vi "MPM_imaging -v5.vi"() -> ()   [LabVIEW 2014]
uses:
  <vilib>/Analysis/baseanly.llb/Mean (DBL).vi
  <vilib>/DAQmx/read.llb/DAQmx Read (Analog 2D DBL NChan NSamp).vi
  <vilib>/DAQmx/read.llb/DAQmx Read (Analog 1D DBL 1Chan NSamp).vi
  <resource>/objmgr/daqmx.rc
  <vilib>/Analysis/NI_AALBase.lvlib
panel:
  out "Integratedfile":string
  out "Rawfile":string
  out "Standard deviationslow":dbl format="%.6f"
  out "Standard deviation fast":dbl format="%.6f"
  out "Mirror error":dbl[][](graph)
  out "Mirrors with offset":dbl[][](graph)
  out "Mirror position":dbl[][](graph)
  out "Samplenumbers":i32
  out "Delay (pixels)":dbl
  out "Galvo Delay (sec)":dbl format="%#_6e"
  out "Xrange":u16
  out "Execution time per loop":dbl[][](graph)
  out "Delay vs output":dbl[][](graph)
  in  "Index (col)":i32
  in  "Length to cut":i32
  in  "Delay increment":dbl=1e-07
  out "Execution time":dbl
  in  "No. of delay iterations":i32=1
  out "Delay vs output":dbl[][](array[numeric])
  out "ms timer":u32
  in  "Line scan on/off (raw)":bool
  in  "Line scan on/off (proccesed)":bool
  in  "Linear/log (integrated)":u16(ring) items=["linear", "log"]
  in  "Linecut direction (fast/slow) (integrated)":u16(ring) items=["fast", "slow"]
  out "Linecut profile (integrted)":dbl[](graph)
  out "Image (integrated)":dbl[][](graph)
  in  "error in (no error)":errorcluster
  out "error out":errorcluster
  out "Linecut profile (raw)":dbl[](graph)
  in  "Linear/Log (raw)":u16(ring) items=["Linear", "Log"]
  in  "Linecut direction (fast/slow) (raw)":u8(ring) items=["fast", "slow"]
  in  "Tab Control":enum32{"Scan and Image", "Save data"}(tab)
  out "Actual (sampling rate/pixel rate)":dbl
  in  "Soft reset after scan":bool
  out "Laser rep. rate (Hz)":dbl
  out "Actual (laser rep. rate/pixel rate)":dbl
  out "Actual pixel rate (Hz)":dbl
  out "Actual line scan rate (Hz)":dbl
  out "Initial sampling rate (Hz)":dbl
  in  "Scan dimension":T1(ring)
  in  "X scan parameters":T2={"Center \n"=0.0, "Scan amplitude"=1.0, "# of pixels"=100}
  in  "Y scan parameters":T3={"Center "=0.0, "Scan amplitude \n"=1.0, "# of pixels"=100}
  in  "Z scan parameters":T4
  out "Actual sampling rate (Hz)":dbl
  out "voltage/degree ratio (V/degree)":dbl
  in  "# of scans":u16(ring) items=["No scan", "Single scan", "Repeated scan"]
  in  "Initial line scan rate (Hz)":dbl(slide)=200.0 scale=0.0..200.0
  in  "Points/pixel":u16=6
  in  "+z":bool
  in  "-z":bool
  in  "Exit the program":bool
  in  "+x":bool
  in  "-x":bool
  in  "+y":bool
  in  "-y":bool
  out "Moving x":bool
  in  "X step":dbl=0.1
  in  "Move X":dbl=14.3034736
  out "Moving y":bool
  in  "Y step":dbl=1.0
  in  "Move Y":dbl=11.6422302
  out "upper z-limit":dbl
  out "lower z-limit":dbl
  out "Moving z":bool
  in  "Z step":dbl=0.001
  in  "Move Z":dbl=18.8888872
  in  "set lower z-limit":dbl
  in  "set upper z-limit":dbl=19.2
  in  "Average in other dim":dbl=1.0
  out "z stack":i32
  out "single (line counter)":i32
  out "Frame rate (s)":dbl format="%.4f"
  out "Time left for stack (s)":dbl format="%#.2g"
  out "lower y-limit":dbl
  out "upper y-limit":dbl
  out "lower x-limit":dbl
  out "upper x-limit":dbl
  in  "set upper y-limit":dbl
  in  "set lower y-limit":dbl
  in  "set upper x-limit":dbl
  in  "set lower x-limit":dbl
  in  "Row by row update?":bool=TRUE
  in  "Stop":bool
  in  "Sample clock source":tag="/Dev1/PFI0"
  in  "Scan mode":T5(ring)=enum."Single Direction (Uniform)"
  out "Theoretical frame rate":dbl format="%_5g"
  in  "Galvomirror delay (sec)":dbl=0.0003 format="%#_6e"
  in  "Lissajous Cluster":cluster{"a":dbl, "b":dbl, "delta":dbl}={"a"=1.0, "b"=2.0, "delta"=0.0} {"delta" format="%_3g"; "b" format="%0.2p"; "a" format="%_3g"}
  in  "Laser rep rate":dbl=120000.0 format="%#_13g"
  out "Galvo speed OK?":bool
  out "Onboard Sample clock?":bool
  in  "Soften":bool
  in  "Asymmetry sawtooth":dbl=0.5
  in  "Sample Clock Delay":dbl=6.7e-06
  in  "Delay from sample clock":bool
  in  "Samp Clk. Delay Units":i32(ring)=10364 items=["Seconds"=10364, "Ticks"=10304]
  in  "Soften points":i32=3
  in  "Track mirror":bool
  out "Pixel Delay":dbl
  in  "File name (integrated). (must end with extension \".txt\")":string="run1_p.txt"
  out "Appended path (integrated)":path
  out "Save tiff stack (integrated)?":bool=TRUE
  out "Auto-save during single scan (integrated)?":bool=TRUE
  out "Save tiff stack (raw)?":bool
  in  "Auto-save during single scan (raw)?":bool=TRUE
  in  "File name (raw). (must end with extension \".txt\")":string="run1_r.txt"
  out "Appended path (raw)":path
  out "Image (raw)":dbl[][](graph)
  # "Controls"
  # "Galvo tracking and\ndelay compensation"
  # "piezo:      0-20   um   \ngalvo: -10 - 10 degrees"
  # "piezo:      0-20   um   \ngalvo: -10 - 10 degrees"
  # "piezo:      0-20   um   \ngalvo: -10 - 10 degrees"
  # "Move sample stage"
  # "Smoothening parameters"
  # "Pattern parameters"
  # "Trigger Delay parameters"
  # "Indicators"
  # "(only for galvomirrors)"
  # "(>=2 when pixel rate is lower than amplifier bandwidth)"
  # "(>=10 )"
  # "(piezo: um/galvo: degree)"
  # "(piezo: um/galvo: degree)"
  # "(>1)"
  # "(piezo: um/galvo: degree)"
  # "(piezo: um/galvo: degree)"
  # "(>1)"
  # "(piezo: um/galvo: degree)"
  # "(piezo: um/galvo: degree)"
  # "(>1)"
  # "Raw"
  # "Pixel integrated"
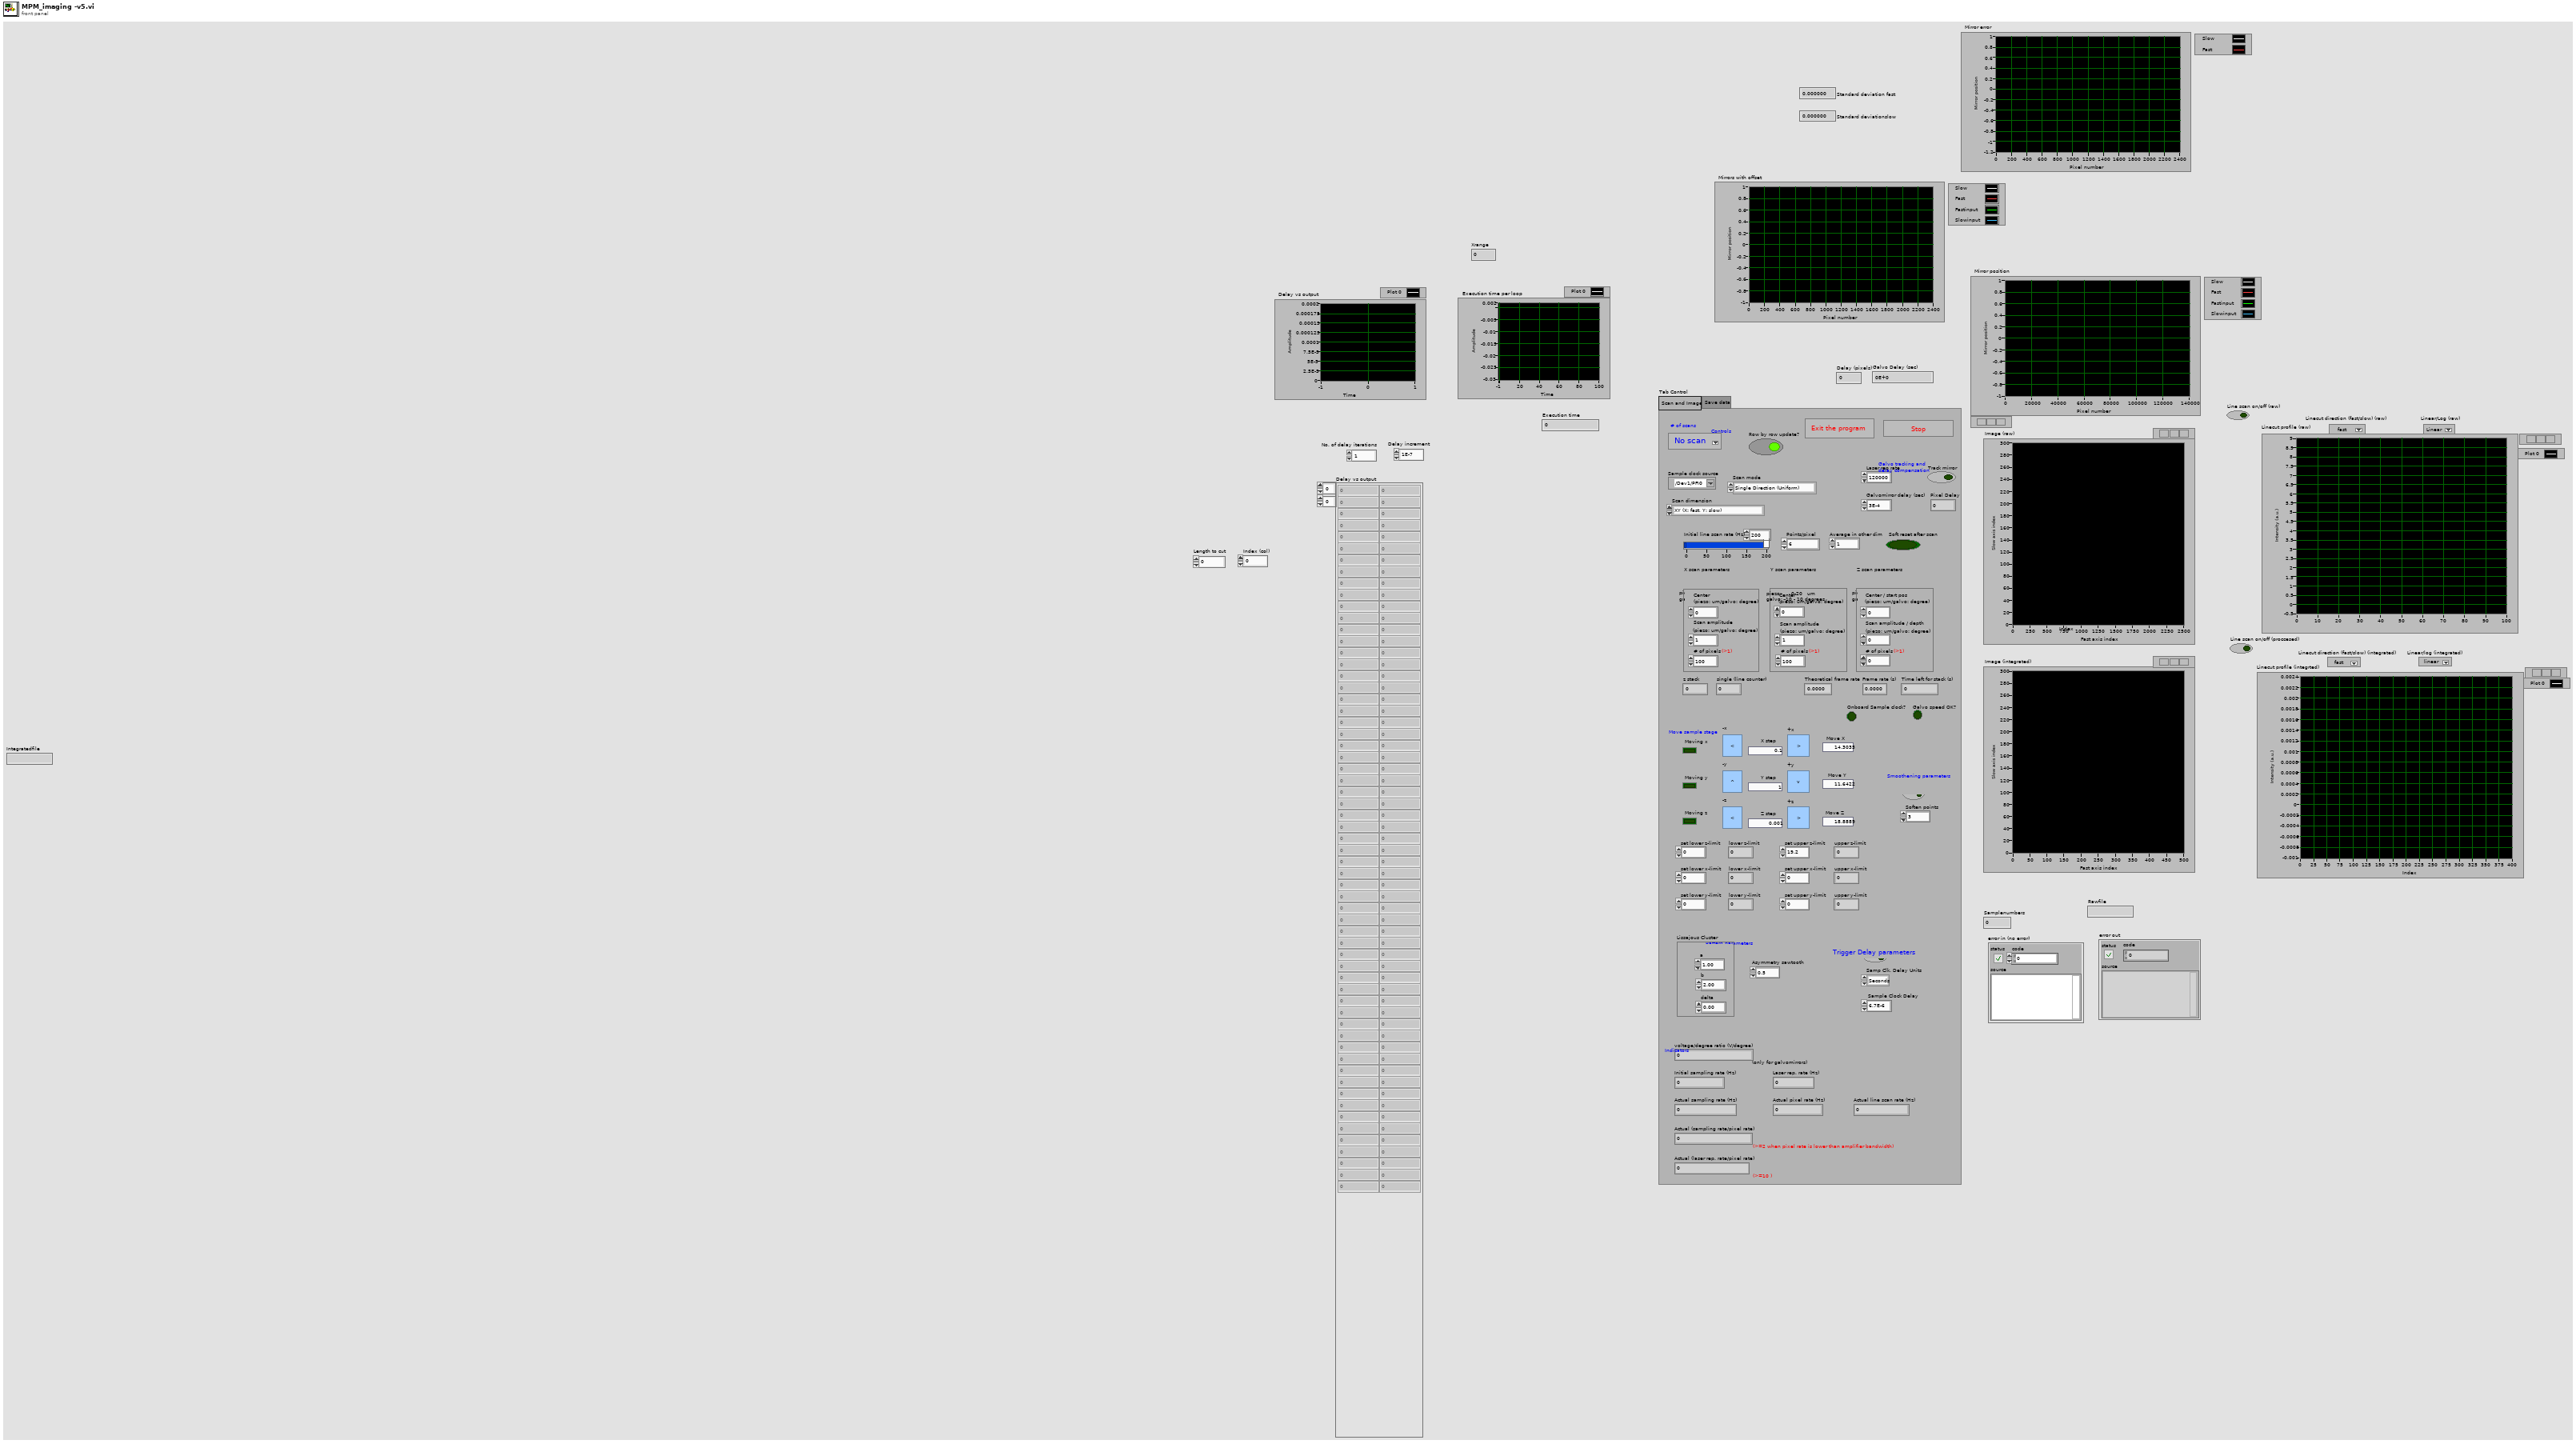
[diagram p1: front panel]
types:
  T1 = enum8{"XY (X: fast, Y: slow)", "XYZ (X: fast, Y: medium, Z: slow)"}
  T2 = cluster{"Center \n":dbl, "Scan amplitude":dbl, "# of pixels":u16}
  T3 = cluster{"Center ":dbl, "Scan amplitude \n":dbl, "# of pixels":u16}
  T4 = cluster{"Center / start pos ":dbl, "Scan amplitude / depth\n":dbl, "# of pixels":u16}
  T5 = enum16{"Lissajous", "Adjustable sawtooth", "Single Direction (Uniform)", "Single Direction (Fast Reset)", "Bi-Directional"}
  T6 = cluster{"VISA resource name":refnum<visa-resource-name>, "Device name":string, "Controller address":i32, "error":errorcluster}
  T7 = cluster{"# of pixels":u16, "Center / start pos ":dbl, "Scan amplitude / depth\n":dbl}
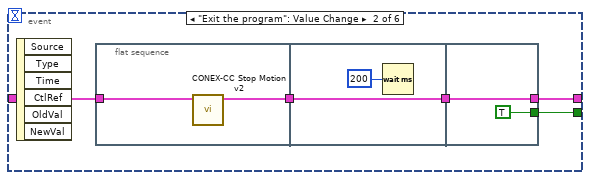
[diagram p2: hidden frame]
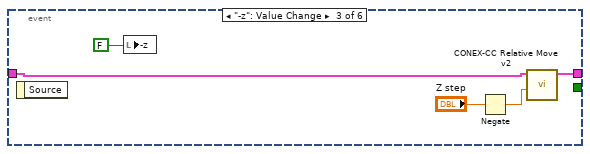
[diagram p3: hidden frame]
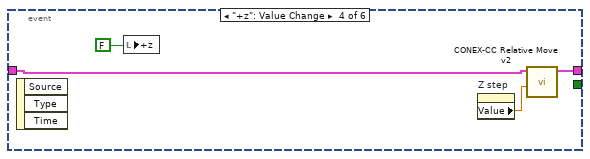
[diagram p4: hidden frame]
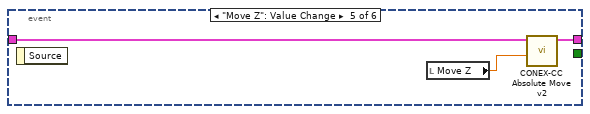
[diagram p5: hidden frame]
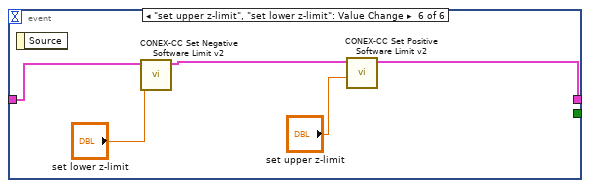
[diagram p6: hidden frame]
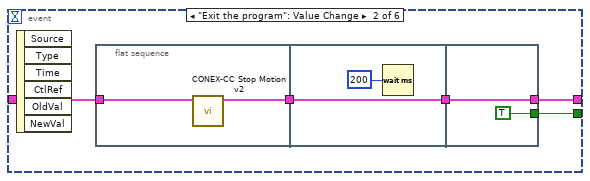
[diagram p7: hidden frame]
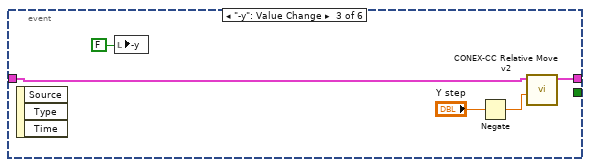
[diagram p8: hidden frame]
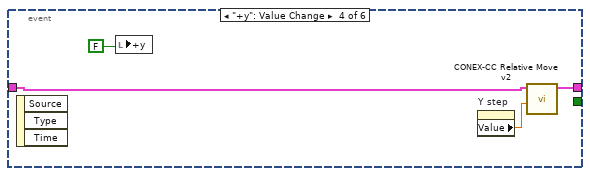
[diagram p9: hidden frame]
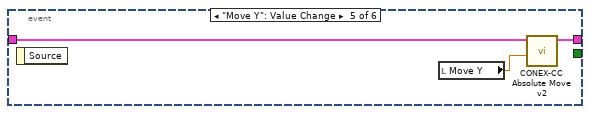
[diagram p10: hidden frame]
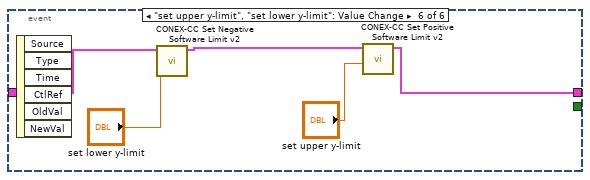
[diagram p11: hidden frame]
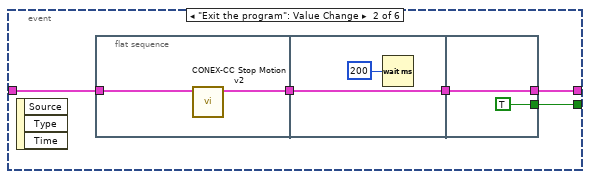
[diagram p12: hidden frame]
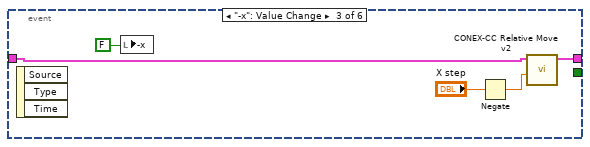
[diagram p13: hidden frame]
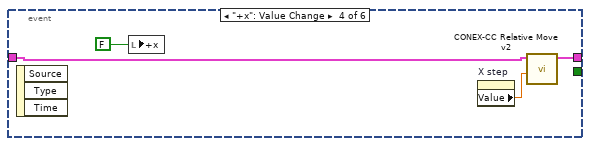
[diagram p14: hidden frame]
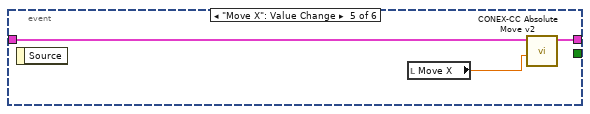
[diagram p15: hidden frame]
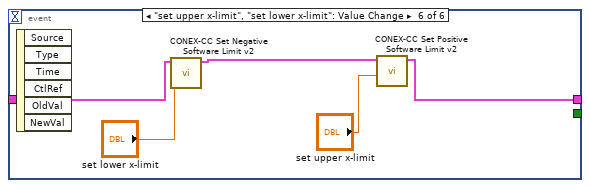
[diagram p16: hidden frame]
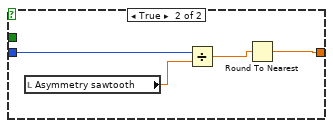
[diagram p18: hidden frame]
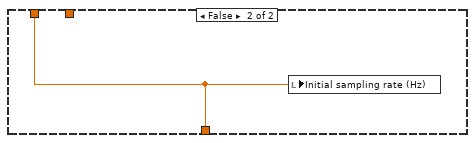
[diagram p19: hidden frame]
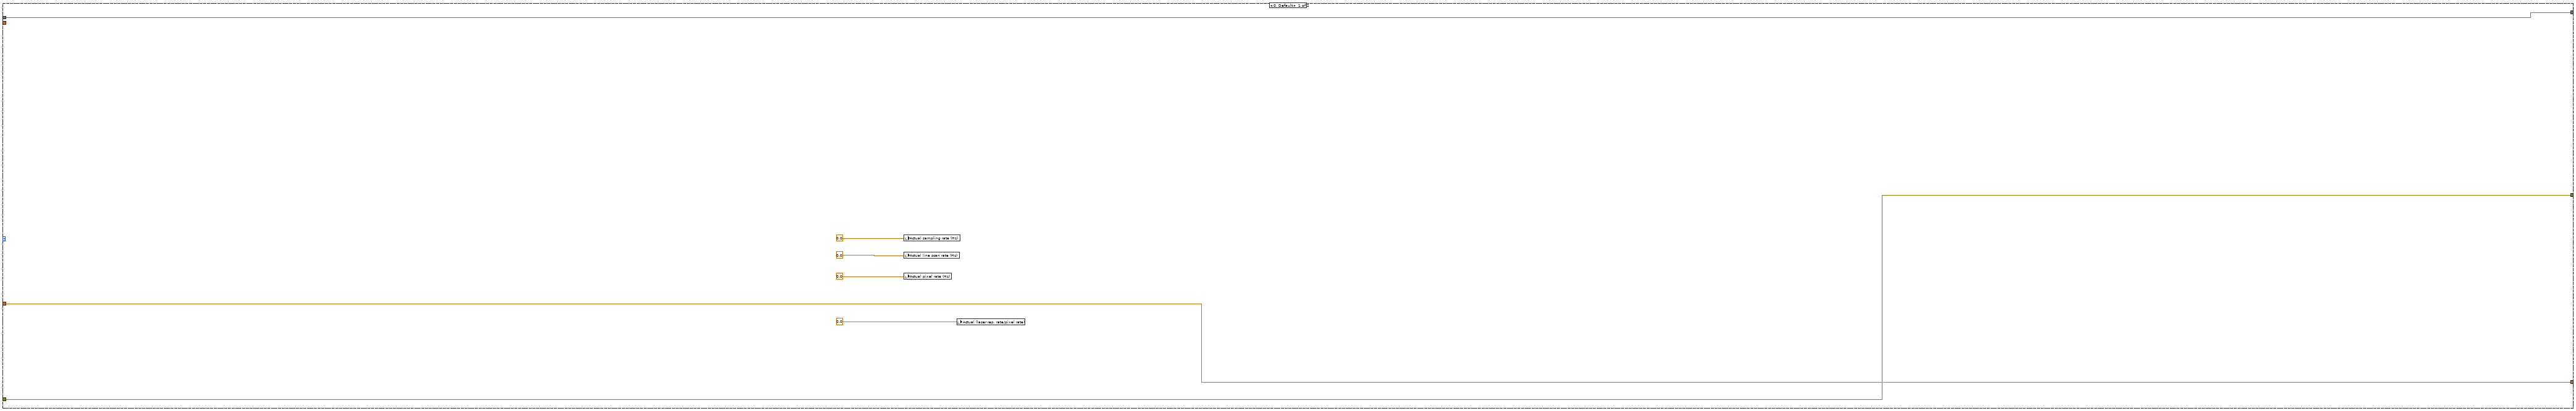
[diagram p20: hidden frame]
diagram:
  w14 = FALSE
  # "There is a physical delay of galvo response (Small Angle Step Response of around 3 microsec) which can be verified in the track mirror option (given by Galvo Delay (sec) and Delay (Pixels)).\nThis delay can be included while taking images in the control 'Galvomirror delay'.  \nGalvomirror delay x  initial sampling rate (laser rep rate for laser as trigger) is the correspong delay in pixel number."
  # "Adjustable sawtooth pattern is controlled by asymmetry sawtooth control. When it is 0.5 the pattern is a triangle. For asymmetry sawtooth =0.9 the pattern becomes single\ndirection fast reset"
  # "Soften is for smoothening the raster pattern.  Twice the number of soften points are added both at the peak and dip. This means in one fast axis cycle 4 x soften points are added."
  # "Sample clock delay is the delay between fluoresecence peak and laser trigger (when sample clock is laser trigger). This delay is varied from 1E-7 (can't be zero) to 8 microsec  in a loop which runs 'no. of delay iterations' times to obtain the maximum signal. The delay is then set to that value.  Delay value depends only on the pre-amp settings and in general lies between 6.8E-6 to 7.5E-6"
  # "0: no scan, 1: single scan, 2: repeat scan"
  # "Newport controls"
  # "only for galvomirrors"
  # "piezo:      0-20   um   \ngalvo: -10 - 10 degrees"
  # "piezo:      0-20   um   \ngalvo: -10 - 10 degrees"
  # "piezo:      0-20   um   \ngalvo: -10 - 10 degrees"
  n1 = local write "-x"(w14) -> ()
  n2 = local write "+x"(w14) -> ()
  n3 = Format Date/Time String(time format string (%c)="%H_%M_%S_") -> (date/time string=w3:string)  [unwired: 2 in]
  n4 = Format Date/Time String(time format string (%c)="%H_%M_%S_") -> (date/time string=w7:string)  [unwired: 2 in]
  n5 = Concatenate Strings(w3, "File name (integrated). (must end with extension \".txt\")") -> (→"Integratedfile":string)
  n6 = call "Connect Newport Instrument_edit.vi"("Numeric"=i8 1, "String"="ASRL4::INSTR") -> ("Device Connection Cluster"=w16:T6)  [unwired: 5 in, 4 out]
  n7 = call "Connect Newport Instrument_edit.vi"("Numeric"=i8 1, "String"="ASRL3::INSTR") -> ("Device Connection Cluster"=w15:T6)  [unwired: 5 in, 4 out]
  n8 = call "Connect Newport Instrument_edit.vi"("Numeric"=i8 1, "String"="ASRL5::INSTR") -> ("Device Connection Cluster"=w9:T6)  [unwired: 5 in, 4 out]
  n9 = Concatenate Strings(w7, "File name (raw). (must end with extension \".txt\")") -> (→"Rawfile":string)
  n10 = while {
    shift-right: [w32] -> w12
    shift-left: w16 -> [w31]
    stop <- w30 stop-if-true
    n11 = event shown="[0] Timeout" {
      selector: _ -> [_ _ _ _ _ _]
      dyn-events: _ -> [_ _ _ _ _ _]
      timeout: 100 -> [_ _ _ _ _ _]
      tunnel: [_ w46 _ _ _ _] -> w30
      tunnel: w31 -> [w44 w47 w57 w63 w67 w69]
      tunnel: [w43 w49 w60 w62 w66 w68] -> w32
      event Timeout {
        n12 = event-data() -> ()  [unwired: 4 out]
        n13 = call "CONEX-CC Get Current Position v2.vi"("Connection Cluster in"=w44) -> ("Current position"=w38:dbl, "Connection Cluster out"=w37:T6)  [unwired: 8 in, 1 out]
        n14 = local write "Move Y"(w38) -> ()
        n15 = Unbundle By Name(w37) -> ("error"=w39:errorcluster)  [unwired: 1 out]
        n16 = call "CONEX-CC Get Negative Software Limit v2.vi"("Connection Cluster in"=w37) -> ("Left limit"=→"lower y-limit":dbl, "Connection Cluster out"=w36:T6)  [unwired: 9 in]
        n17 = call "CONEX-CC Get Positive Software Limit v2.vi"("Connection Cluster in"=w36) -> ("Right limit"=→"upper y-limit":dbl, "Connection Cluster out"=w35:T6)  [unwired: 9 in]
        n18 = local write "error out"(w39) -> ()
        n19 = call "CONEX-CC Get Positioner Error And Controller State v2.vi"("Connection Cluster in"=w35) -> ("Controller state"=w42:string, "Connection Cluster out"=w43:T6)  [unwired: 8 in, 1 out]
        n20 = Equal?(x="28" ("y"), y=w42) -> (x = y?=→"Moving y":bool)
      }
      event "Exit the program": Value Change {
        n21 = event-data() -> ()  [unwired: 7 out]
        n22 = flat-sequence {
          tunnel: [w51] -> w45
          tunnel: w47 -> [w50]
          tunnel: w45 -> [w53]
          tunnel: [w53] -> w48
          tunnel: [w55] -> w49
          tunnel: w48 -> [w55]
          tunnel: [TRUE] -> w46
          frame #0 {
            n23 = call "CONEX-CC Stop Motion v2.vi"("Connection Cluster in"=w50) -> ("Connection Cluster out"=w51:T6)  [unwired: 10 in]
          }
          frame #1 {
            n24 = Wait (ms)(milliseconds to wait=u32 200 ("attente (ms)")) -> ()  [unwired: 1 out]
          }
          frame #2 {
          }
        }
      }
      event "-y": Value Change {
        n25 = event-data() -> ()  [unwired: 4 out]
        n26 = local write "-y"(FALSE ("-")) -> ()
        n27 = Negate(x="Y step") -> (-x=w58:dbl)
        n28 = call "CONEX-CC Relative Move v2.vi"("Relative displacement"=w58, "Connection Cluster in"=w57) -> ("Connection Cluster out"=w60:T6)  [unwired: 9 in]
      }
      event "+y": Value Change {
        n29 = event-data() -> ()  [unwired: 4 out]
        n30 = local write "+y"(FALSE ("+")) -> ()
        n31 = property on="Y step" class="DigNum (strict)"() -> ("Value"=w64:dbl)  [unwired: 2 in, 2 out]
        n32 = call "CONEX-CC Relative Move v2.vi"("Relative displacement"=w64, "Connection Cluster in"=w63) -> ("Connection Cluster out"=w62:T6)  [unwired: 9 in]
      }
      event "Move Y": Value Change {
        n33 = event-data() -> ()  [unwired: 2 out]
        n34 = local read "Move Y"() -> (w65:dbl)
        n35 = call "CONEX-CC Absolute Move v2.vi"("Target position"=w65, "Connection Cluster in"=w67) -> ("Connection Cluster out"=w66:T6)  [unwired: 5 in, 2 out]
      }
      event "set upper y-limit", "set lower y-limit": Value Change {
        n36 = event-data() -> ()  [unwired: 7 out]
        n37 = call "CONEX-CC Set Negative Software Limit v2.vi"("Negative limit (left)"="set lower y-limit", "Connection Cluster in"=w69) -> ("Connection Cluster out"=w72:T6)  [unwired: 9 in]
        n38 = call "CONEX-CC Set Positive Software Limit v2.vi"("Positive limit (right)"="set upper y-limit", "Connection Cluster in"=w72) -> ("Connection Cluster out"=w68:T6)  [unwired: 9 in]
      }
    }
  }
  n39 = while {
    shift-right: [w76] -> w11
    shift-left: w9 -> [w75]
    stop <- w74 stop-if-true
    n40 = event shown="[0] Timeout" {
      selector: _ -> [_ _ _ _ _ _]
      dyn-events: _ -> [_ _ _ _ _ _]
      timeout: 100 -> [_ _ _ _ _ _]
      tunnel: [_ w90 _ _ _ _] -> w74
      tunnel: w75 -> [w88 w91 w101 w107 w111 w116]
      tunnel: [w87 w93 w104 w106 w110 w114] -> w76
      event Timeout {
        n41 = event-data() -> ()  [unwired: 4 out]
        n42 = call "CONEX-CC Get Current Position v2.vi"("Connection Cluster in"=w88) -> ("Current position"=w77:dbl, "Connection Cluster out"=w83:T6)  [unwired: 8 in, 1 out]
        n43 = local write "Move Z"(w77) -> ()
        n44 = Unbundle By Name(w83) -> ("error"=w78:errorcluster)  [unwired: 1 out]
        n45 = call "CONEX-CC Get Negative Software Limit v2.vi"("Connection Cluster in"=w83) -> ("Left limit"=→"lower z-limit":dbl, "Connection Cluster out"=w82:T6)  [unwired: 9 in]
        n46 = call "CONEX-CC Get Positive Software Limit v2.vi"("Connection Cluster in"=w82) -> ("Right limit"=→"upper z-limit":dbl, "Connection Cluster out"=w81:T6)  [unwired: 9 in]
        n47 = local write "error out"(w78) -> ()
        n48 = call "CONEX-CC Get Positioner Error And Controller State v2.vi"("Connection Cluster in"=w81) -> ("Controller state"=w86:string, "Connection Cluster out"=w87:T6)  [unwired: 8 in, 1 out]
        n49 = Equal?(x=w86, y="28") -> (x = y?=→"Moving z":bool)
      }
      event "Exit the program": Value Change {
        n50 = event-data() -> ()  [unwired: 7 out]
        n51 = flat-sequence {
          tunnel: [w95] -> w89
          tunnel: w91 -> [w94]
          tunnel: w89 -> [w97]
          tunnel: [w97] -> w92
          tunnel: [w99] -> w93
          tunnel: w92 -> [w99]
          tunnel: [TRUE] -> w90
          frame #0 {
            n52 = call "CONEX-CC Stop Motion v2.vi"("Connection Cluster in"=w94) -> ("Connection Cluster out"=w95:T6)  [unwired: 10 in]
          }
          frame #1 {
            n53 = Wait (ms)(milliseconds to wait=u32 200 ("attente (ms)")) -> ()  [unwired: 1 out]
          }
          frame #2 {
          }
        }
      }
      event "-z": Value Change {
        n54 = event-data() -> ()  [unwired: 2 out]
        n55 = local write "-z"(FALSE ("-")) -> ()
        n56 = Negate(x="Z step") -> (-x=w102:dbl)
        n57 = call "CONEX-CC Relative Move v2.vi"("Relative displacement"=w102, "Connection Cluster in"=w101) -> ("Connection Cluster out"=w104:T6)  [unwired: 9 in]
      }
      event "+z": Value Change {
        n58 = event-data() -> ()  [unwired: 4 out]
        n59 = local write "+z"(FALSE ("+")) -> ()
        n60 = property on="Z step" class="DigNum (strict)"() -> ("Value"=w108:dbl)  [unwired: 2 in, 2 out]
        n61 = call "CONEX-CC Relative Move v2.vi"("Relative displacement"=w108, "Connection Cluster in"=w107) -> ("Connection Cluster out"=w106:T6)  [unwired: 9 in]
      }
      event "Move Z": Value Change {
        n62 = event-data() -> ()  [unwired: 2 out]
        n63 = local read "Move Z"() -> (w109:dbl)
        n64 = call "CONEX-CC Absolute Move v2.vi"("Target position"=w109, "Connection Cluster in"=w111) -> ("Connection Cluster out"=w110:T6)  [unwired: 5 in, 2 out]
      }
      event "set upper z-limit", "set lower z-limit": Value Change {
        n65 = event-data() -> ()  [unwired: 2 out]
        n66 = call "CONEX-CC Set Negative Software Limit v2.vi"("Negative limit (left)"="set lower z-limit", "Connection Cluster in"=w116) -> ("Connection Cluster out"=w115:T6)  [unwired: 9 in]
        n67 = call "CONEX-CC Set Positive Software Limit v2.vi"("Positive limit (right)"="set upper z-limit", "Connection Cluster in"=w115) -> ("Connection Cluster out"=w114:T6)  [unwired: 9 in]
      }
    }
  }
  n68 = while {
    shift-right: [w120] -> w13
    shift-left: w15 -> [w119]
    stop <- w118 stop-if-true
    n69 = event shown="[0] Timeout" {
      selector: _ -> [_ _ _ _ _ _]
      dyn-events: _ -> [_ _ _ _ _ _]
      timeout: 100 -> [_ _ _ _ _ _]
      tunnel: [_ w134 _ _ _ _] -> w118
      tunnel: w119 -> [w132 w135 w145 w151 w155 w157]
      tunnel: [w131 w137 w148 w150 w154 w156] -> w120
      event Timeout {
        n70 = event-data() -> ()  [unwired: 4 out]
        n71 = call "CONEX-CC Get Current Position v2.vi"("Connection Cluster in"=w132) -> ("Current position"=w126:dbl, "Connection Cluster out"=w125:T6)  [unwired: 8 in, 1 out]
        n72 = local write "Move X"(w126) -> ()
        n73 = Unbundle By Name(w125) -> ("error"=w127:errorcluster)  [unwired: 1 out]
        n74 = call "CONEX-CC Get Negative Software Limit v2.vi"("Connection Cluster in"=w125) -> ("Left limit"=→"lower x-limit":dbl, "Connection Cluster out"=w124:T6)  [unwired: 9 in]
        n75 = call "CONEX-CC Get Positive Software Limit v2.vi"("Connection Cluster in"=w124) -> ("Right limit"=→"upper x-limit":dbl, "Connection Cluster out"=w123:T6)  [unwired: 9 in]
        n76 = local write "error out"(w127) -> ()
        n77 = call "CONEX-CC Get Positioner Error And Controller State v2.vi"("Connection Cluster in"=w123) -> ("Controller state"=w130:string, "Connection Cluster out"=w131:T6)  [unwired: 8 in, 1 out]
        n78 = Equal?(x=w130, y="28") -> (x = y?=→"Moving x":bool)
      }
      event "Exit the program": Value Change {
        n79 = event-data() -> ()  [unwired: 4 out]
        n80 = flat-sequence {
          tunnel: [w139] -> w133
          tunnel: w135 -> [w138]
          tunnel: w133 -> [w141]
          tunnel: [w141] -> w136
          tunnel: [w143] -> w137
          tunnel: w136 -> [w143]
          tunnel: [TRUE] -> w134
          frame #0 {
            n81 = call "CONEX-CC Stop Motion v2.vi"("Connection Cluster in"=w138) -> ("Connection Cluster out"=w139:T6)  [unwired: 10 in]
          }
          frame #1 {
            n82 = Wait (ms)(milliseconds to wait=u32 200 ("attente (ms)")) -> ()  [unwired: 1 out]
          }
          frame #2 {
          }
        }
      }
      event "-x": Value Change {
        n83 = event-data() -> ()  [unwired: 4 out]
        n84 = local write "-x"(FALSE ("-")) -> ()
        n85 = Negate(x="X step") -> (-x=w146:dbl)
        n86 = call "CONEX-CC Relative Move v2.vi"("Relative displacement"=w146, "Connection Cluster in"=w145) -> ("Connection Cluster out"=w148:T6)  [unwired: 9 in]
      }
      event "+x": Value Change {
        n87 = event-data() -> ()  [unwired: 4 out]
        n88 = local write "+x"(FALSE ("+")) -> ()
        n89 = property on="X step" class="DigNum (strict)"() -> ("Value"=w152:dbl)  [unwired: 2 in, 2 out]
        n90 = call "CONEX-CC Relative Move v2.vi"("Relative displacement"=w152, "Connection Cluster in"=w151) -> ("Connection Cluster out"=w150:T6)  [unwired: 9 in]
      }
      event "Move X": Value Change {
        n91 = event-data() -> ()  [unwired: 2 out]
        n92 = local read "Move X"() -> (w153:dbl)
        n93 = call "CONEX-CC Absolute Move v2.vi"("Target position"=w153, "Connection Cluster in"=w155) -> ("Connection Cluster out"=w154:T6)  [unwired: 5 in, 2 out]
      }
      event "set upper x-limit", "set lower x-limit": Value Change {
        n94 = event-data() -> ()  [unwired: 7 out]
        n95 = call "CONEX-CC Set Negative Software Limit v2.vi"("Negative limit (left)"="set lower x-limit", "Connection Cluster in"=w157) -> ("Connection Cluster out"=w160:T6)  [unwired: 9 in]
        n96 = call "CONEX-CC Set Positive Software Limit v2.vi"("Positive limit (right)"="set upper x-limit", "Connection Cluster in"=w160) -> ("Connection Cluster out"=w156:T6)  [unwired: 9 in]
      }
    }
  }
  n97 = while {
    tunnel: w9 -> [w200]
    tunnel: [w199] -> w10
    stop <- "Exit the program" stop-if-true
    # "For Case II above clock sampling rate is independent of initial line\nscan rate. Laser rep rate is the sampling rate."
    # "a:  Laser rep rate: points/sec\nb:  X scan #of pixels x points/pixel: points/line\nCase I: When sample clock source is the laser trigger\nline scan rate is a/b which should always be less than 200 Hz\n(maximum freq. of galvo)\nTherefore b > laser rep rate/200\nCase II: When sample clock source is DAQ onboard clock, the galvo freq.\nis independent of laser rep. rate and ia given by initial line scan rate\n(set by user with maximum value as 200)"
    # "Maximum galvo rate"
    # "Actual line scan rate \nwith laser trigger as sample clock"
    n98 = local read "X scan parameters"() -> (w186:T2)
    n99 = local read "Scan mode"() -> (w166:T5)
    n100 = Unbundle By Name(w186) -> ("# of pixels"=w163:u16)
    n101 = Equal?(x=w166, y=T5."Adjustable sawtooth") -> (x = y?=w164:bool)
    n102 = Equal?(x=w166, y=T5."Single Direction (Fast Reset)") -> (x = y?=w161:bool)
    n103 = case shown="False" w164 {
      tunnel: w163 -> [w202 w211]
      tunnel: [w201 w209] -> w162
      tunnel: w161 -> [w203 _]
      frame False {
        n104 = case shown="True" w203 {
          tunnel: w202 -> [w204 w207]
          tunnel: [w204 w205] -> w201
          frame False {
          }
          frame True {
            n105 = Divide(x=w207, y=0.9) -> (x/y=w206:dbl)
            n106 = Round To Nearest(number=w206) -> (nearest integer value=w205:dbl)
          }
        }
      }
      frame True {
        n107 = local read "Asymmetry sawtooth"() -> (w212:dbl)
        n108 = Divide(x=w211, y=w212) -> (x/y=w210:dbl)
        n109 = Round To Nearest(number=w210) -> (nearest integer value=w209:dbl)
      }
    }
    n110 = local read "Onboard Sample clock?"() -> (w176:bool)
    n111 = local read "error in (no error)"() -> (w174:errorcluster)
    n112 = local read "Initial sampling rate (Hz)"() -> (w168:dbl)
    n113 = local write "Sample Clock Delay"("Sample Clock Delay") -> ()
    n114 = local read "Sample clock source"() -> (w188:tag)
    n115 = local read "Points/pixel"() -> (w187:u16)
    n116 = Multiply(x=w187, y=w162) -> (x*y=w177:dbl)
    n117 = case shown="True" w176 {
      tunnel: w177 -> [w215 _]
      tunnel: "Laser rep rate" -> [_ w216]
      tunnel: [w213 w216] -> w172
      frame True {
        n118 = local read "Initial line scan rate (Hz)"() -> (w214:dbl)
        n119 = Multiply(x=w215, y=w214) -> (x*y=w213:dbl)
        n120 = local write "Initial sampling rate (Hz)"(w213) -> ()
      }
      frame False {
        n121 = local write "Initial sampling rate (Hz)"(w216) -> ()
      }
    }
    n122 = Not Equal?(x=w188, y=tag "/Dev1/PFI0") -> (x != y?=w179:bool)
    "Onboard Sample clock?" <- w179
    n123 = Divide(x=w168, y=w177) -> (x/y=w180:dbl)
    n124 = local read "Y scan parameters"() -> (w185:T3)
    n125 = Divide(x="Laser rep rate", y=ext 200.0) -> (x/y=w181:ext)
    n126 = Greater Or Equal?(x=w177, y=w181) -> (x >= y?=w178:bool)
    n127 = Reciprocal(x=w172) -> (1/x=w170:dbl)
    n128 = Unbundle By Name(w185) -> ("# of pixels"=w184:u16)
    n129 = Or(x=w179, y=w178) -> (x .or. y?=→"Galvo speed OK?":bool)
    n130 = Divide(x="Galvomirror delay (sec)", y=w170) -> (x/y=→"Pixel Delay":dbl)
    n131 = Divide(x=w184, y=w180) -> (x/y=→"Theoretical frame rate":dbl)
    n132 = Initialize Array(0.0 ("element"), 100 ("dimension size"), 2 ("dimension size")) -> (w193:dbl[][])
    n133 = for {
      N: "No. of delay iterations" -> [_]
      tunnel: w174 -> [w228]
      tunnel: w200 -> [w225]
      tunnel: [w224] -> w199
      shift-right: [w220] -> _
      shift-left: "Sample Clock Delay" -> [w219]
      tunnel: [w223] -> _ mode=indexing
      tunnel: w193 -> [w223] mode=indexing
      tunnel: [w222] -> w192 mode=indexing
      n134 = call "Time Delay"("error in (no error)"=w228, "Delay Time (s)"=0.1) -> ("error out"=w227:errorcluster)  [unwired: 9 in]
      n135 = local read "# of scans"() -> (w229:u16)
      n136 = case shown="1, 2" w229 {
        tunnel: w227 -> [w236 w267]
        tunnel: [w236 w256] -> w224
        tunnel: w225 -> [_ w260]
        tunnel: w219 -> [w231 w246]
        tunnel: [w231 w252] -> w218
        tunnel: w223 -> [w230 w251]
        tunnel: w219 -> [_ w250]
        tunnel: [w230 w249] -> w222
        tunnel: "Stop" -> [_ w245]
        frame 0, Default {
          n137 = local write "Actual sampling rate (Hz)"(0.0) -> ()
          n138 = local write "Actual line scan rate (Hz)"(0.0) -> ()
          n139 = local write "Actual pixel rate (Hz)"(0.0) -> ()
          n140 = local write "Actual (laser rep. rate/pixel rate)"(0.0) -> ()
        }
        frame 1, 2 {
          w274 = 1.0
          n141 = local read "Y scan parameters"() -> (w280:T3)
          n142 = local read "Scan mode"() -> (w241:T5)
          n143 = local read "X scan parameters"() -> (w285:T2)
          n144 = local read "Z scan parameters"() -> (w275:T4)
          n145 = local write "voltage/degree ratio (V/degree)"(w274) -> ()
          n146 = Unbundle By Name(w275) -> ("Center / start pos"=w261:dbl, "Scan amplitude / depth"=w247:dbl, "# of pixels"=w268:u16)
          n147 = Unbundle By Name(w280) -> ("Center"=w279:dbl, "Scan amplitude"=w278:dbl, "# of pixels"=w269:u16)
          n148 = Unbundle By Name(w285) -> ("Center"=w284:dbl, "Scan amplitude"=w283:dbl, "# of pixels"=w242:u16)
          n149 = Equal?(x=w241, y=T5."Adjustable sawtooth") -> (x = y?=w243:bool)
          n150 = Equal?(x=w241, y=T5."Single Direction (Fast Reset)") -> (x = y?=w239:bool)
          n151 = case shown="True" w243 {
            tunnel: w242 -> [w287 w295]
            tunnel: [w286 w293] -> w238
            tunnel: w239 -> [w288 _]
            frame False {
              n152 = case shown="False" w288 {
                tunnel: w287 -> [w289 w291]
                tunnel: [w289 w290] -> w286
                frame False {
                }
                frame True {
                  n153 = Divide(x=w291, y=0.9) -> (x/y=w290:dbl)
                }
              }
            }
            frame True {
              n154 = local read "Asymmetry sawtooth"() -> (w294:dbl)
              n155 = Divide(x=w295, y=w294) -> (x/y=w293:dbl)
            }
          }
          n156 = Add(x=w284, y=w283) -> (x+y=w282:dbl)
          n157 = Subtract(x=w284, y=w283) -> (x-y=w281:dbl)
          n158 = Add(x=w279, y=w278) -> (x+y=w277:dbl)
          n159 = Subtract(x=w279, y=w278) -> (x-y=w276:dbl)
          n160 = Multiply(x=w274, y=w282) -> (x*y=w273:dbl)
          n161 = Multiply(x=w274, y=w281) -> (x*y=w272:dbl)
          n162 = Multiply(x=w274, y=w277) -> (x*y=w271:dbl)
          n163 = Multiply(x=w274, y=w276) -> (x*y=w270:dbl)
          n164 = Round To Nearest(number=w238) -> (nearest integer value=w237:dbl)
          n165 = while {
            tunnel: w273 -> [w437]
            tunnel: w272 -> [w436]
            tunnel: w271 -> [w434]
            tunnel: w270 -> [w433]
            tunnel: w237 -> [w435]
            tunnel: w269 -> [w432]
            tunnel: w261 -> [w431]
            tunnel: w247 -> [w430]
            tunnel: w268 -> [w386]
            tunnel: w267 -> [w426]
            tunnel: [w420] -> w266
            tunnel: [w417] -> w265
            tunnel: [w416] -> w264
            tunnel: [w385] -> w263
            tunnel: [w359] -> w262
            tunnel: [w411] -> w254
            tunnel: w260 -> [w409]
            tunnel: [w408] -> w259
            tunnel: w246 -> [w347]
            tunnel: [w364] -> w252
            tunnel: w251 -> [w399]
            tunnel: w250 -> [w398]
            tunnel: [w397] -> w249
            tunnel: w245 -> [w361]
            i -> [w366]
            stop <- w408 stop-if-true
            # "For saving scan parameters"
            # "single"
            # "DAQ movement"
            # "z stack counter"
            n166 = local read "Scan dimension"() -> (w438:T1)
            n167 = Increment(x=w366) -> (x+1=w404:i32)
            n168 = local write "z stack"(w404) -> ()
            n169 = case shown="\"XYZ (X: fast, Y: medium, Z: slow)\"" w438 {
              tunnel: w437 -> [w1163 w1213]
              tunnel: w436 -> [w1164 w1214]
              tunnel: w435 -> [w1173 w1208]
              tunnel: w434 -> [w1161 w1211]
              tunnel: w433 -> [w1162 w1212]
              tunnel: w432 -> [w1174 w1221]
              tunnel: w431 -> [w1182 w1206]
              tunnel: w430 -> [w1181 w1203]
              tunnel: w386 -> [w1180 w1228]
              tunnel: w366 -> [_ w1227]
              tunnel: [w1175 w1222] -> w341
              tunnel: [w1174 w1221] -> w357
              tunnel: [w1178 w1225] -> w429
              tunnel: [w1177 w1224] -> w428
              tunnel: [w1176 cluster{u8, dbl, dbl} {1, 0.0, 0.0}] -> w427
              tunnel: w426 -> [w1179 w1226]
              tunnel: [w1179 w1226] -> w418
              tunnel: [w1173 w1208] -> w410
              tunnel: [w1160 w1210] -> w417
              tunnel: w409 -> [_ w1207]
              tunnel: w347 -> [w1152 w1184]
              tunnel: [w1152 w1184] -> w352
              frame "XY (X: fast, Y: slow)", Default {
                w1153 = "\r\n"
                w1158 = "um "
                w1156 = "um-"
                w1172 = 50.0
                n170 = local read "Points/pixel"() -> (w1159:u16)
                n171 = Multiply(x=w1164, y=w1172) -> (x*y=w1171:dbl)
                n172 = Multiply(x=w1163, y=w1172) -> (x*y=w1170:dbl)
                n173 = Multiply(x=w1173, y=w1159) -> (x*y=w1183:dbl)
                n174 = Multiply(x=w1162, y=w1172) -> (x*y=w1169:dbl)
                n175 = Multiply(x=w1161, y=w1172) -> (x*y=w1168:dbl)
                n176 = To Unsigned Word Integer(number=w1183) -> (unsigned 16bit integer=w1175:u16)
                "Xrange" <- w1175
                n177 = Number To Decimal String(number=w1170) -> (decimal integer string=w1165:string)  [unwired: 1 in]
                n178 = Number To Decimal String(number=w1171) -> (decimal integer string=w1166:string)  [unwired: 1 in]
                n179 = Number To Decimal String(number=w1169) -> (decimal integer string=w1155:string)  [unwired: 1 in]
                n180 = Number To Decimal String(number=w1168) -> (decimal integer string=w1157:string)  [unwired: 1 in]
                n181 = Bundle(w1175, w1163, w1164) -> (w1178:cluster{u16, dbl, dbl})  [unwired: 1 in]
                n182 = Bundle("# of pixels"=w1174, w1161, w1162) -> (w1177:cluster{"# of pixels":u16, dbl, dbl})  [unwired: 1 in]
                n183 = Bundle("# of pixels"=w1180, "Center / start pos"=w1182, "Scan amplitude / depth"=w1181) -> (w1176:T7)  [unwired: 1 in]
                n184 = Concatenate Strings("X: ", w1166, w1156, w1165, w1158, w1153, "Y: ", w1155, w1156, w1157, w1158, w1153) -> (w1160:string)
              }
              frame "XYZ (X: fast, Y: medium, Z: slow)" {
                w1190 = "\r\n"
                w1194 = "um "
                w1198 = "um-"
                w1215 = 50.0
                n185 = local read "Points/pixel"() -> (w1209:u16)
                n186 = Decrement(x=w1228) -> (x-1=w1186:u16)
                n187 = Divide(x=w1203, y=w1186) -> (x/y=w1185:dbl)
                n188 = Equal?(x=0.0, y=w1227) -> (x = y?=w1188:bool)
                n189 = case shown="True" w1188 {
                  tunnel: w1206 -> [_ w1239]
                  tunnel: w1185 -> [w1231 _]
                  tunnel: w1207 -> [w1230 w1238]
                  frame False {
                    n190 = call "CONEX-CC Relative Move v2.vi"("Relative displacement"=w1231, "Connection Cluster in"=w1230) -> ("Connection Cluster out"=w1232:T6)  [unwired: 9 in]
                    n191 = while {
                      tunnel: w1232 -> [w1235]
                      stop <- w1233 stop-if-true
                      n192 = call "CONEX-CC Get Current Position v2.vi"("Connection Cluster in"=w1235) -> ("Connection Cluster out"=w1234:T6)  [unwired: 8 in, 2 out]
                      n193 = call "CONEX-CC Get Positioner Error And Controller State v2.vi"("Connection Cluster in"=w1234) -> ("Controller state"=w1237:string)  [unwired: 8 in, 2 out]
                      n194 = Not Equal?(x=w1237, y="28") -> (x != y?=w1233:bool)
                    }
                  }
                  frame True {
                    n195 = call "CONEX-CC Absolute Move v2.vi"("Target position"=w1239, "Connection Cluster in"=w1238) -> ("Connection Cluster out"=w1240:T6)  [unwired: 5 in, 2 out]
                    n196 = while {
                      tunnel: w1240 -> [w1243]
                      stop <- w1241 stop-if-true
                      n197 = call "CONEX-CC Get Current Position v2.vi"("Connection Cluster in"=w1243) -> ("Connection Cluster out"=w1242:T6)  [unwired: 8 in, 2 out]
                      n198 = call "CONEX-CC Get Positioner Error And Controller State v2.vi"("Connection Cluster in"=w1242) -> ("Controller state"=w1245:string)  [unwired: 8 in, 2 out]
                      n199 = Not Equal?(x=w1245, y="28") -> (x != y?=w1241:bool)
                    }
                  }
                }
                n200 = Multiply(x=w1208, y=w1209) -> (x*y=w1229:dbl)
                n201 = Multiply(x=w1214, y=w1215) -> (x*y=w1220:dbl)
                n202 = Multiply(x=w1213, y=w1215) -> (x*y=w1219:dbl)
                n203 = Multiply(x=w1212, y=w1215) -> (x*y=w1218:dbl)
                n204 = Multiply(x=w1211, y=w1215) -> (x*y=w1217:dbl)
                n205 = Multiply(x=w1203, y=1000.0) -> (x*y=w1205:dbl)
                n206 = To Unsigned Word Integer(number=w1229) -> (unsigned 16bit integer=w1222:u16)
                n207 = Number To Decimal String(number=w1219) -> (decimal integer string=w1216:string)  [unwired: 1 in]
                n208 = Number To Decimal String(number=w1220) -> (decimal integer string=w1197:string)  [unwired: 1 in]
                n209 = Number To Decimal String(number=w1218) -> (decimal integer string=w1200:string)  [unwired: 1 in]
                n210 = Number To Decimal String(number=w1217) -> (decimal integer string=w1195:string)  [unwired: 1 in]
                n211 = Number To Decimal String(number=w1206) -> (decimal integer string=w1192:string)  [unwired: 1 in]
                n212 = Number To Decimal String(number=w1205) -> (decimal integer string=w1201:string)  [unwired: 1 in]
                n213 = Bundle(w1222, w1213, w1214) -> (w1225:cluster{u16, dbl, dbl})  [unwired: 1 in]
                n214 = Bundle("# of pixels"=w1221, w1211, w1212) -> (w1224:cluster{"# of pixels":u16, dbl, dbl})  [unwired: 1 in]
                n215 = Concatenate Strings("X: ", w1197, w1198, w1216, w1194, w1190, "Y: ", w1200, w1198, w1195, w1194, w1190, "Z start_pos: ", w1192, "mm" ("string"), w1190, "Z depth:     " ("string"), w1201, "um" ("string"), w1190) -> (w1210:string)
              }
            }
            n216 = local read "Scan mode"() -> (w419:T5)
            n217 = local read "Galvo speed OK?"() -> (w362:bool)
            n218 = case shown="False" "Track mirror" {
              tunnel: [w464 w505] -> w442
              tunnel: w429 -> [w463 w504]
              tunnel: w428 -> [w462 w503]
              tunnel: w427 -> [w461 w502]
              tunnel: w418 -> [w460 w501]
              tunnel: [w459 w500] -> w396
              tunnel: [w458 w499] -> w387
              tunnel: w352 -> [w457 w498]
              tunnel: [w456 w497] -> w363
              tunnel: w362 -> [w455 w496]
              tunnel: [w454 w495] -> w360
              tunnel: [w453 w494] -> w349
              frame True {
                n219 = case shown="False" w455 {
                  tunnel: [refnum<k21> refnum ("task out") w493] -> w464
                  tunnel: [errorcluster {"status"=FALSE, "code"=0, "source"=""} ("error out") w492] -> w454
                  tunnel: w463 -> [_ w491]
                  tunnel: w462 -> [_ w490]
                  tunnel: w461 -> [_ w489]
                  tunnel: w460 -> [_ w488]
                  tunnel: [0.0 ("Actual sample rate (Hz)") w484] -> w456
                  tunnel: w457 -> [_ w485]
                  tunnel: [refnum<k21> refnum ("task out") w487] -> w459
                  tunnel: [errorcluster {"status"=FALSE, "code"=0, "source"=""} ("error out") w486] -> w458
                  tunnel: [dbl[][] [] ("Waveform Graph") w473] -> _
                  tunnel: [dbl[][] [] ("Waveform Graph") w473] -> w453
                  frame False {
                  }
                  frame True {
                    n220 = local read "Initial sampling rate (Hz)"() -> (w483:dbl)
                    n221 = local read "Lissajous Cluster"() -> (w476:cluster{"a":dbl, "b":dbl, "delta":dbl})
                    n222 = local read "Soften"() -> (w474:bool)
                    n223 = local read "Soft reset after scan"() -> (w482:bool)
                    n224 = local read "Asymmetry sawtooth"() -> (w475:dbl)
                    n225 = local read "Scan mode"() -> (w477:T5)
                    n226 = local read "Soften points"() -> (w472:i32)
                    n227 = local read "Samp Clk. Delay Units"() -> (w478:i32)
                    n228 = local read "Sample clock source"() -> (w480:tag)
                    n229 = call "Scan_setup.vi"("X axis"=w491, "Y axis"=w490, "Z axis"=w489, "Initial sample rate (Hz)"=w483, "error in (no error)"=w488, "Scan mode"=w477, "Sample clock source"=w480, "Lissajous Cluster"=w476, "Home the stage after scan?"=w482, "asymmetry"=w475, "Soften"=w474, "Soften points"=w472) -> ("task out"=w487:refnum<k21>, "Waveform Graph"=w473:dbl[][], "Samples per channel"=w481:i32, "Actual sample rate (Hz)"=w484:dbl, "error out"=w492:errorcluster)  [unwired: 11 in]
                    n230 = local read "Delay from sample clock"() -> (w479:bool)
                    n231 = call "Galvo_track.vi"("Samples per channel"=w481, "Sample rate (Hz)"=w484, "error in (no error)"=w488, "Samp Clk. Delay Units"=w478, "Sample Clock Delay"=w485, "Sample clock source"=w480, "Delay from sample clock"=w479) -> ("task out"=w493:refnum<k21>, "error out"=w486:errorcluster)  [unwired: 19 in]
                  }
                }
              }
              frame False {
                n232 = case shown="True" w496 {
                  tunnel: [refnum<k21> refnum ("task out") w533] -> w505
                  tunnel: [errorcluster {"status"=FALSE, "code"=0, "source"=""} ("error out") w532] -> w495
                  tunnel: w504 -> [_ w531]
                  tunnel: w503 -> [_ w530]
                  tunnel: w502 -> [_ w529]
                  tunnel: w501 -> [_ w528]
                  tunnel: [0.0 ("Actual sample rate (Hz)") w524] -> w497
                  tunnel: w498 -> [_ w525]
                  tunnel: [refnum<k21> refnum ("task out") w527] -> w500
                  tunnel: [errorcluster {"status"=FALSE, "code"=0, "source"=""} ("error out") w526] -> w499
                  tunnel: [dbl[][] [] ("Waveform Graph") w513] -> w494
                  frame False {
                  }
                  frame True {
                    n233 = local read "Initial sampling rate (Hz)"() -> (w523:dbl)
                    n234 = local read "Lissajous Cluster"() -> (w516:cluster{"a":dbl, "b":dbl, "delta":dbl})
                    n235 = local read "Soften"() -> (w514:bool)
                    n236 = local read "Soft reset after scan"() -> (w522:bool)
                    n237 = local read "Asymmetry sawtooth"() -> (w515:dbl)
                    n238 = local read "Scan mode"() -> (w517:T5)
                    n239 = local read "Samp Clk. Delay Units"() -> (w518:i32)
                    n240 = local read "Sample clock source"() -> (w520:tag)
                    n241 = call "Scan_setup.vi"("X axis"=w531, "Y axis"=w530, "Z axis"=w529, "Initial sample rate (Hz)"=w523, "error in (no error)"=w528, "Scan mode"=w517, "Sample clock source"=w520, "Lissajous Cluster"=w516, "Home the stage after scan?"=w522, "asymmetry"=w515, "Soften"=w514, "Soften points"="Soften points") -> ("task out"=w527:refnum<k21>, "Waveform Graph"=w513:dbl[][], "Samples per channel"=w521:i32, "Actual sample rate (Hz)"=w524:dbl, "error out"=w532:errorcluster)  [unwired: 11 in]
                    n242 = local read "Delay from sample clock"() -> (w519:bool)
                    n243 = call "Detector_setup.vi"("Samples per channel"=w521, "Sample rate (Hz)"=w524, "error in (no error)"=w528, "Samp Clk. Delay Units"=w518, "Sample Clock Delay"=w525, "Sample clock source"=w520, "Delay from sample clock"=w519) -> ("task out"=w533:refnum<k21>, "error out"=w526:errorcluster)  [unwired: 19 in]
                  }
                }
              }
            }
            n244 = case shown="\"Single Direction (Fast Reset)\", Default" w419 {
              tunnel: [w1064 w1083 w1102 w1121 w1140] -> w416
              frame "Single Direction (Fast Reset)", Default {
                w1052 = "\r\n"
                w1059 = "Hz; "
                n245 = local read "Average in other dim"() -> (w1055:dbl)
                n246 = local read "Points/pixel"() -> (w1056:u16)
                n247 = local read "Actual sampling rate (Hz)"() -> (w1067:dbl)
                n248 = local read "Actual line scan rate (Hz)"() -> (w1065:dbl)
                n249 = local read "Actual pixel rate (Hz)"() -> (w1066:dbl)
                n250 = Number To Decimal String(number=w1056) -> (decimal integer string=w1053:string)  [unwired: 1 in]
                n251 = Number To Decimal String(number=w1055) -> (decimal integer string=w1050:string)  [unwired: 1 in]
                n252 = Number To Decimal String(number=w1067) -> (decimal integer string=w1058:string)  [unwired: 1 in]
                n253 = Number To Decimal String(number=w1066) -> (decimal integer string=w1061:string)  [unwired: 1 in]
                n254 = Number To Decimal String(number=w1065) -> (decimal integer string=w1063:string)  [unwired: 1 in]
                n255 = Concatenate Strings("single direction fast reset; ", w1052, "sample rate: ", w1058, w1059, w1052, "pixel rate: ", w1061, w1059, w1052, "line scan rate rate: ", w1063, w1059, w1052, "Points per pixel: " ("string"), w1053, w1052, "Average in other dim.: " ("string"), w1050) -> (w1064:string)
              }
              frame "Adjustable sawtooth" {
                w1071 = "\r\n"
                w1078 = "Hz; "
                n256 = local read "Average in other dim"() -> (w1074:dbl)
                n257 = local read "Points/pixel"() -> (w1075:u16)
                n258 = local read "Actual sampling rate (Hz)"() -> (w1086:dbl)
                n259 = local read "Actual line scan rate (Hz)"() -> (w1084:dbl)
                n260 = local read "Actual pixel rate (Hz)"() -> (w1085:dbl)
                n261 = Number To Decimal String(number=w1075) -> (decimal integer string=w1072:string)  [unwired: 1 in]
                n262 = Number To Decimal String(number=w1074) -> (decimal integer string=w1069:string)  [unwired: 1 in]
                n263 = Number To Decimal String(number=w1086) -> (decimal integer string=w1077:string)  [unwired: 1 in]
                n264 = Number To Decimal String(number=w1085) -> (decimal integer string=w1080:string)  [unwired: 1 in]
                n265 = Number To Decimal String(number=w1084) -> (decimal integer string=w1082:string)  [unwired: 1 in]
                n266 = Concatenate Strings("Adjustable sawtooth;", w1071, "sample rate: ", w1077, w1078, w1071, "pixel rate: ", w1080, w1078, w1071, "line scan rate rate: ", w1082, w1078, w1071, "Points per pixel: " ("string"), w1072, w1071, "Average in other dim.: " ("string"), w1069) -> (w1083:string)
              }
              frame "Lissajous" {
                w1090 = "\r\n"
                w1097 = "Hz; "
                n267 = local read "Average in other dim"() -> (w1093:dbl)
                n268 = local read "Points/pixel"() -> (w1094:u16)
                n269 = local read "Actual sampling rate (Hz)"() -> (w1105:dbl)
                n270 = local read "Actual line scan rate (Hz)"() -> (w1103:dbl)
                n271 = local read "Actual pixel rate (Hz)"() -> (w1104:dbl)
                n272 = Number To Decimal String(number=w1094) -> (decimal integer string=w1091:string)  [unwired: 1 in]
                n273 = Number To Decimal String(number=w1093) -> (decimal integer string=w1088:string)  [unwired: 1 in]
                n274 = Number To Decimal String(number=w1105) -> (decimal integer string=w1096:string)  [unwired: 1 in]
                n275 = Number To Decimal String(number=w1104) -> (decimal integer string=w1099:string)  [unwired: 1 in]
                n276 = Number To Decimal String(number=w1103) -> (decimal integer string=w1101:string)  [unwired: 1 in]
                n277 = Concatenate Strings("\"Lissajous\";", w1090, "sample rate: ", w1096, w1097, w1090, "pixel rate: ", w1099, w1097, w1090, "line scan rate rate: ", w1101, w1097, w1090, "Points per pixel: " ("string"), w1091, w1090, "Average in other dim.: " ("string"), w1088) -> (w1102:string)
              }
              frame "Single Direction (Uniform)" {
                w1109 = "\r\n"
                w1116 = "Hz; "
                n278 = local read "Average in other dim"() -> (w1113:dbl)
                n279 = local read "Points/pixel"() -> (w1112:u16)
                n280 = local read "Actual sampling rate (Hz)"() -> (w1122:dbl)
                n281 = local read "Actual line scan rate (Hz)"() -> (w1124:dbl)
                n282 = local read "Actual pixel rate (Hz)"() -> (w1123:dbl)
                n283 = Number To Decimal String(number=w1112) -> (decimal integer string=w1107:string)  [unwired: 1 in]
                n284 = Number To Decimal String(number=w1113) -> (decimal integer string=w1110:string)  [unwired: 1 in]
                n285 = Number To Decimal String(number=w1122) -> (decimal integer string=w1115:string)  [unwired: 1 in]
                n286 = Number To Decimal String(number=w1123) -> (decimal integer string=w1118:string)  [unwired: 1 in]
                n287 = Number To Decimal String(number=w1124) -> (decimal integer string=w1120:string)  [unwired: 1 in]
                n288 = Concatenate Strings("single direction uniform; ", w1109, "sample rate: ", w1115, w1116, w1109, "pixel rate: ", w1118, w1116, w1109, "line scan rate rate: ", w1120, w1116, w1109, "Average in other dim.: " ("string"), w1110, w1109, "points/pixel: " ("string"), w1107) -> (w1121:string)
              }
              frame "Bi-Directional" {
                w1129 = "\r\n"
                w1135 = "Hz; "
                n289 = local read "Actual sampling rate (Hz)"() -> (w1143:dbl)
                n290 = local read "Actual line scan rate (Hz)"() -> (w1141:dbl)
                n291 = local read "Actual pixel rate (Hz)"() -> (w1142:dbl)
                n292 = local read "Points/pixel"() -> (w1132:u16)
                n293 = Number To Decimal String(number=w1132) -> (decimal integer string=w1130:string)  [unwired: 1 in]
                n294 = Number To Decimal String(number=w1143) -> (decimal integer string=w1134:string)  [unwired: 1 in]
                n295 = Number To Decimal String(number=w1142) -> (decimal integer string=w1137:string)  [unwired: 1 in]
                n296 = Number To Decimal String(number=w1141) -> (decimal integer string=w1139:string)  [unwired: 1 in]
                n297 = local read "Average in other dim"() -> (w1127:dbl)
                n298 = Number To Decimal String(number=w1127) -> (decimal integer string=w1126:string)  [unwired: 1 in]
                n299 = Concatenate Strings("bi-direction; ", w1129, "sample rate: ", w1134, w1135, w1129, "pixel rate: ", w1137, w1135, w1129, "line scan rate rate: ", w1139, w1135, w1129, "points/pixel: " ("string"), w1130, w1129, "Average in other dim.: " ("string"), w1126) -> (w1140:string)
              }
            }
            n300 = local read "Laser rep. rate (Hz)"() -> (w422:dbl)
            n301 = Divide(x=w363, y=w341) -> (x/y=w425:dbl)
            n302 = local write "Actual sampling rate (Hz)"(w363) -> ()
            n303 = local write "Actual line scan rate (Hz)"(w425) -> ()
            n304 = Multiply(x=w425, y=w410) -> (x*y=w414:dbl)
            n305 = Divide(x=w422, y=w414) -> (x/y=w421:dbl)
            n306 = local write "Actual pixel rate (Hz)"(w414) -> ()
            n307 = local write "Actual (laser rep. rate/pixel rate)"(w421) -> ()
            n308 = Divide(x=w363, y=w414) -> (x/y=w415:dbl)
            n309 = local write "Actual (sampling rate/pixel rate)"(w415) -> ()
            n310 = Index Array(array=w349, index (row)=0) -> (element=w354:dbl[])  [unwired: 1 in]
            n311 = Array Size(array=w354) -> (size(s)=→"Samplenumbers":i32)
            n312 = Threshold 1D Array(2:0.0 ("threshold y"), 3:w354) -> (0:w348:dbl)  [unwired: 1 in]
            n313 = local read "Soften points"() -> (w345:i32)
            n314 = local read "Soften"() -> (w343:bool)
            n315 = Multiply(x=w345, y=2.0) -> (x*y=w344:dbl)
            n316 = local read "Row by row update?"() -> (w340:bool)
            n317 = local read "Y scan parameters"() -> (w389:T3)
            n318 = call <vilib>:"DAQmx Start Task.vi"("task/channels in"=w442, "error in"=w387) -> ("task out"=w439:refnum<k21>, "error out"=w440:errorcluster)  [unwired: 12 in]
            n319 = Merge Errors(w360, w440) -> (w370:errorcluster)
            n320 = case shown="True" w343 {
              tunnel: w344 -> [_ w448]
              tunnel: w341 -> [w444 w447]
              tunnel: [w444 w446] -> w342
              tunnel: w340 -> [_ w445]
              frame False {
              }
              frame True {
                n321 = case shown="False" w445 {
                  tunnel: w448 -> [_ w452]
                  tunnel: w447 -> [w449 w451]
                  tunnel: [w449 w450] -> w446
                  frame False {
                  }
                  frame True {
                    n322 = Add(x=w452, y=w451) -> (x+y=w450:dbl)
                  }
                }
              }
            }
            n323 = local read "Row by row update?"() -> (w390:bool)
            n324 = call <vilib>:"DAQmx Start Task.vi"("task/channels in"=w396, "error in"=w370) -> ("task out"=w441:refnum<k21>, "error out"=w356:errorcluster)  [unwired: 12 in]
            n325 = Unbundle By Name(w389) -> ("# of pixels"=w388:u16)
            n326 = Initialize Array(0.0, w357, w341) -> (w391:dbl[][])
            n327 = Initialize Array(0.0 ("element"), 100 ("dimension size"), 2 ("dimension size")) -> (w392:dbl[][])
            n328 = case shown="False" w390 {
              tunnel: w391 -> [w572 _]
              tunnel: w441 -> [w571 w765]
              tunnel: w356 -> [w570 w793]
              tunnel: w439 -> [w569 w792]
              tunnel: w342 -> [w568 w788]
              tunnel: [w556 w791] -> w412
              tunnel: [w567 w765] -> w365
              tunnel: [w566 w790] -> w411
              tunnel: [w554 w785] -> w407
              tunnel: w352 -> [w565 w771]
              tunnel: [w555 w771] -> w364
              tunnel: [w564 w785] -> w384
              tunnel: w392 -> [w562 _]
              tunnel: w388 -> [_ w789]
              tunnel: w357 -> [_ w787]
              tunnel: w341 -> [_ w786]
              tunnel: w357 -> [w563 _]
              tunnel: [w559 w785] -> w378
              tunnel: [w558 w784] -> w377
              tunnel: [w557 w784] -> w375
              tunnel: w361 -> [w553 w770]
              tunnel: w349 -> [w552 w769]
              tunnel: w348 -> [_ w767]
              frame True {
                n329 = while {
                  shift-right: [w576] -> _
                  shift-left: w572 -> [w624]
                  tunnel: [w603] -> w567
                  tunnel: [w615] -> w556
                  tunnel: w571 -> [w603]
                  tunnel: w570 -> [w625]
                  tunnel: w569 -> [w614]
                  tunnel: w568 -> [w588]
                  tunnel: w563 -> [w596]
                  tunnel: [w623] -> w566
                  tunnel: w565 -> [w616]
                  tunnel: [w616] -> w555
                  tunnel: [w600] -> w564
                  shift-right: [w611] -> _
                  shift-left: _ -> [w612]
                  tunnel: w562 -> [w610] mode=indexing
                  tunnel: [w609] -> w561 mode=indexing
                  tunnel: [w600] -> w559
                  tunnel: [w601] -> w558
                  tunnel: [w601] -> w557
                  tunnel: [w600] -> w554
                  tunnel: w553 -> [w598]
                  tunnel: w552 -> [w594]
                  i -> [w592]
                  stop <- w602 stop-if-true
                  # "row-by-row update"
                  # "2D images"
                  n330 = Equal To 0?(x=w592) -> (x = 0?=w589:bool)
                  n331 = case shown="True" w589 {
                    tunnel: w588 -> [w725 w728]
                    tunnel: [w725 w726] -> w591
                    frame False {
                    }
                    frame True {
                      n332 = local read "Pixel Delay"() -> (w727:dbl)
                      n333 = Add(x=w727, y=w728) -> (x+y=w726:dbl)
                    }
                  }
                  n334 = local read "Track mirror"() -> (w597:bool)
                  n335 = case shown="False" w597 {
                    tunnel: [w737 w744] -> w627
                    tunnel: w625 -> [w736 w743]
                    tunnel: w614 -> [w735 w742]
                    tunnel: w591 -> [_ w741]
                    tunnel: [w734 w740] -> w608
                    tunnel: [dbl[] [] ("data") w739] -> w590
                    tunnel: [w729 dbl[][] [] ("data")] -> w595
                    frame True {
                      n336 = local read "Samplenumbers"() -> (w732:i32)
                      n337 = call-poly <vilib>:"DAQmx Read.vi"("task/channels in"=w735, "number of samples per channel"=w732, "error in"=w736) -> ("task out"=w734:refnum<k21>, "data"=w730:dbl[][], "error out"=w737:errorcluster)  [unwired: 10 in]
                      n338 = Multiply(x=w730, y=2.0) -> (x*y=w729:dbl[][])
                    }
                    frame False {
                      n339 = call-poly <vilib>:"DAQmx Read.vi"("task/channels in"=w742, "number of samples per channel"=w741, "error in"=w743) -> ("task out"=w740:refnum<k21>, "data"=w739:dbl[], "error out"=w744:errorcluster)  [unwired: 10 in]
                    }
                  }
                  n340 = case shown="True" w589 {
                    tunnel: w590 -> [w720 w724]
                    tunnel: [w720 w721] -> w575
                    frame False {
                    }
                    frame True {
                      n341 = local read "Pixel Delay"() -> (w722:dbl)
                      n342 = Delete From Array(array=w724, length=w722, index=0) -> (array with subset deleted=w721:dbl[])  [unwired: 1 out]
                    }
                  }
                  n343 = Get Date/Time In Seconds() -> (seconds since 1Jan1904=w611:timestamp)
                  n344 = Equal?(x=w592, y=0) -> (x = y?=w620:bool)
                  n345 = local read "Soften points"() -> (w581:i32)
                  n346 = case shown="True" w620 {
                    frame False {
                    }
                    frame True {
                      n347 = Tick Count (ms)() -> (millisecond timer value=w761:u32)
                      n348 = local write "ms timer"(w761) -> ()
                    }
                  }
                  n349 = Multiply(x=w581, y=2) -> (x*y=w578:i32)
                  n350 = Array Size(array=w575) -> (size(s)=w579:i32)
                  n351 = Subtract(x=w579, y=w578) -> (x-y=w577:i32)
                  n352 = local read "Soften"() -> (w573:bool)
                  n353 = Subtract(x=w612, y=w611) -> (x-y=w599:dbl)
                  "Execution time" <- w599
                  n354 = case shown="True" w573 {
                    tunnel: w578 -> [_ w634]
                    tunnel: w577 -> [_ w633]
                    tunnel: w575 -> [w630 w632]
                    tunnel: [w630 w631] -> w574
                    frame False {
                    }
                    frame True {
                      n355 = Delete From Array(array=w632, length=w634, index=w633) -> (array with subset deleted=w631:dbl[])  [unwired: 1 out]
                    }
                  }
                  n356 = local read "Scan mode"() -> (w587:T5)
                  n357 = Build Array (concatenate)(w595, w594) -> (w593:dbl[][])
                  n358 = local write "Mirror position"(w593) -> ()
                  n359 = case shown="\"Adjustable sawtooth\"" w587 {
                    tunnel: w574 -> [w640 w652 w664 w678 w700]
                    tunnel: w624 -> [w641 w653 w665 w679 w701]
                    tunnel: w592 -> [w637 w649 w661 w677 w697]
                    tunnel: [w639 w651 w663 w671 w699] -> w576
                    tunnel: w596 -> [w636 w648 w660 w674 w696]
                    tunnel: [1.0 ("y") 1.0 ("y") 1.0 ("y") 2.0 ("y") 1.0 ("y")] -> w617
                    frame "Single Direction (Fast Reset)", Default {
                      n360 = Less?(x=w637, y=w636) -> (x < y?=w638:bool)
                      n361 = case shown="True" w638 {
                        tunnel: w641 -> [w642 w646]
                        tunnel: w640 -> [_ w643]
                        tunnel: [w642 w645] -> w639
                        tunnel: w637 -> [_ w644]
                        frame False {
                        }
                        frame True {
                          n362 = Replace Array Subset(array=w646, new element=w643, index (row)=w644) -> (w645:dbl[][])  [unwired: 1 in]
                        }
                      }
                    }
                    frame "Adjustable sawtooth" {
                      n363 = Less?(x=w649, y=w648) -> (x < y?=w650:bool)
                      n364 = case shown="True" w650 {
                        tunnel: w653 -> [w654 w658]
                        tunnel: w652 -> [_ w657]
                        tunnel: [w654 w656] -> w651
                        tunnel: w649 -> [_ w655]
                        frame False {
                        }
                        frame True {
                          n365 = Replace Array Subset(array=w658, new element=w657, index (row)=w655) -> (w656:dbl[][])  [unwired: 1 in]
                        }
                      }
                    }
                    frame "Lissajous" {
                      n366 = Less?(x=w661, y=w660) -> (x < y?=w662:bool)
                      n367 = case shown="True" w662 {
                        tunnel: w665 -> [w666 w670]
                        tunnel: w664 -> [_ w669]
                        tunnel: [w666 w668] -> w663
                        tunnel: w661 -> [_ w667]
                        frame False {
                        }
                        frame True {
                          n368 = Replace Array Subset(array=w670, new element=w669, index (row)=w667) -> (w668:dbl[][])  [unwired: 1 in]
                        }
                      }
                    }
                    frame "Single Direction (Uniform)" {
                      n369 = Multiply(x=w674, y=2) -> (x*y=w675:i32)
                      n370 = Less?(x=w677, y=w675) -> (x < y?=w676:bool)
                      n371 = case shown="True" w676 {
                        tunnel: w677 -> [_ w684]
                        tunnel: w679 -> [w680 w683]
                        tunnel: [w680 w682] -> w671
                        tunnel: w678 -> [_ w681]
                        frame False {
                        }
                        frame True {
                          n372 = Quotient & Remainder(x=w684, y=2) -> (x-y*floor(x/y)=w688:i32, floor(x/y)=w685:i32)
                          n373 = Equal?(x=0, y=w688) -> (x = y?=w686:bool)
                          n374 = case shown="True" w686 {
                            tunnel: w685 -> [_ w694]
                            tunnel: w683 -> [w690 w693]
                            tunnel: [w690 w692] -> w682
                            tunnel: w681 -> [_ w691]
                            frame False {
                            }
                            frame True {
                              n375 = Replace Array Subset(array=w693, new element=w691, index (row)=w694) -> (w692:dbl[][])  [unwired: 1 in]
                            }
                          }
                        }
                      }
                    }
                    frame "Bi-Directional" {
                      n376 = Less?(x=w697, y=w696) -> (x < y?=w698:bool)
                      n377 = case shown="True" w698 {
                        tunnel: w701 -> [w702 w706]
                        tunnel: w700 -> [_ w705]
                        tunnel: [w702 w704] -> w699
                        tunnel: w697 -> [_ w703]
                        frame False {
                        }
                        frame True {
                          n378 = Quotient & Remainder(x=w703, y=2) -> (x-y*floor(x/y)=w709:i32)  [unwired: 1 out]
                          n379 = Equal?(x=0, y=w709) -> (x = y?=w707:bool)
                          n380 = case shown="False" w707 {
                            tunnel: w706 -> [w715 w718]
                            tunnel: [w714 w717] -> w704
                            tunnel: w705 -> [w712 w719]
                            tunnel: w703 -> [w713 w716]
                            frame False {
                              n381 = Reverse 1D Array(array=w712) -> (reversed array=w711:dbl[])
                              n382 = Replace Array Subset(array=w715, new element=w711, index (row)=w713) -> (w714:dbl[][])  [unwired: 1 in]
                            }
                            frame True {
                              n383 = Replace Array Subset(array=w718, new element=w719, index (row)=w716) -> (w717:dbl[][])  [unwired: 1 in]
                            }
                          }
                        }
                      }
                    }
                  }
                  n384 = Multiply(x=w596, y=w617) -> (x*y=w619:dbl)
                  n385 = Decrement(x=w619) -> (x-1=w613:dbl)
                  n386 = Equal?(x=w592, y=w613) -> (x = y?=w618:bool)
                  n387 = call <vilib>:"DAQmx Is Task Done.vi"("task/channels in"=w608, "error in"=w627) -> ("task out"=w607:refnum<k21>, "task done?"=w628:bool, "error out"=w606:errorcluster)  [unwired: 11 out]
                  n388 = case shown="True" w618 {
                    frame False {
                    }
                    frame True {
                      n389 = local read "ms timer"() -> (w760:u32)
                      n390 = Tick Count (ms)() -> (millisecond timer value=w759:u32)
                      n391 = Subtract(x=w759, y=w760) -> (x-y=w757:u32)
                      n392 = Divide(x=w757, y=1000.0) -> (x/y=w756:dbl)
                      n393 = local write "Frame rate (s)"(w756) -> ()
                    }
                  }
                  n394 = property class="DAQmx Read" props=["TotalSampPerChanAcquired", "AvailSampPerChan"](reference=w607, error in=w606) -> (reference out=w615:refnum<k21>, error out=w601:errorcluster, "AvailSampPerChan"=w605:u32)  [unwired: 1 out]
                  n395 = local read "X scan parameters"() -> (w585:T2)
                  n396 = Replace Array Subset(array=w610, new element #1=w599, index #1=w599, new element #2=w592) -> (w609:dbl[])  [unwired: 1 in]
                  n397 = Transpose 2D Array(2D array=w576) -> (transposed array=w586:dbl[][])
                  n398 = local read "Scan mode"() -> (w604:T5)
                  n399 = Equal To 0?(x=w605) -> (x = 0?=w629:bool)
                  n400 = local read "Points/pixel"() -> (w583:u16)
                  n401 = Unbundle By Name(w585) -> ("# of pixels"=w584:u16)
                  n402 = Multiply(x=w584, y=w583) -> (x*y=w582:u16)
                  n403 = case shown="\"Single Direction (Fast Reset)\"" w604 {
                    tunnel: w586 -> [w745 w749 w753 w754 w755]
                    tunnel: [w745 w747 w751 w754 w755] -> w600
                    tunnel: w582 -> [_ w746 w750 _ _]
                    frame "Single Direction (Uniform)", Default {
                    }
                    frame "Single Direction (Fast Reset)" {
                      n404 = Array Subset(array=w749, index (row)=0 ("index"), length (row)=w746) -> (w747:dbl[][])  [unwired: 2 in]
                    }
                    frame "Adjustable sawtooth" {
                      n405 = Array Subset(array=w753, index (row)=0 ("index"), length (row)=w750) -> (w751:dbl[][])  [unwired: 2 in]
                    }
                    frame "Bi-Directional" {
                    }
                    frame "Lissajous" {
                    }
                  }
                  n406 = Unbundle By Name(w627) -> ("status"=w622:bool)
                  n407 = And(x=w629, y=w628) -> (x .and. y?=w626:bool)
                  n408 = Compound Arithmetic op=OR(w626, w622, w598) -> (w602:bool)
                  n409 = Compound Arithmetic op=OR(w622, w598) -> (w623:bool)
                  n410 = local write "Image (raw)"(w600) -> ()
                  "single (line counter)" <- w592
                }
                n411 = Transpose 2D Array(2D array=w561) -> (transposed array=→"Execution time per loop":dbl[][])
              }
              frame False {
                # "2D images"
                n412 = flat-sequence {
                  tunnel: w786 -> [w797]
                  tunnel: w787 -> [w798]
                  tunnel: w788 -> [w799]
                  tunnel: w789 -> [w800]
                  tunnel: w792 -> [w801]
                  tunnel: w793 -> [w802]
                  tunnel: [w802] -> w783
                  tunnel: [w801] -> w782
                  tunnel: [w800] -> w781
                  tunnel: [w799] -> w780
                  tunnel: [w798] -> w779
                  tunnel: [w797] -> w778
                  tunnel: [w796] -> w772
                  tunnel: w769 -> [w795]
                  tunnel: [w795] -> w768
                  tunnel: w767 -> [w794]
                  tunnel: [w794] -> w766
                  tunnel: w783 -> [w843]
                  tunnel: w782 -> [w844]
                  tunnel: w781 -> [w873]
                  tunnel: w780 -> [w872]
                  tunnel: w779 -> [w871]
                  tunnel: w778 -> [w870]
                  tunnel: [w875] -> w777
                  tunnel: [w874] -> w776
                  tunnel: [w869] -> w775
                  tunnel: [w845] -> w774
                  tunnel: [w855] -> w773
                  tunnel: w772 -> [w855]
                  tunnel: w770 -> [w854]
                  tunnel: w768 -> [w833]
                  tunnel: w766 -> [w838]
                  tunnel: [w814] -> w764
                  tunnel: [w1026] -> w784
                  tunnel: [w1027] -> w785
                  tunnel: [w1028] -> w790
                  tunnel: [w1029] -> w791
                  tunnel: w777 -> [w1029]
                  tunnel: w776 -> [w1028]
                  tunnel: w775 -> [w1027]
                  tunnel: w774 -> [w1026]
                  tunnel: w773 -> [w1024]
                  frame #0 {
                    n413 = Get Date/Time In Seconds() -> (seconds since 1Jan1904=w796:timestamp)
                  }
                  frame #1 {
                    n414 = local read "Samplenumbers"() -> (w825:i32)
                    n415 = local read "Galvo speed OK?"() -> (w842:bool)
                    n416 = local read "Pixel Delay"() -> (w828:dbl)
                    n417 = case shown="True" w842 {
                      tunnel: w844 -> [_ w886]
                      tunnel: w843 -> [_ w885]
                      tunnel: w825 -> [_ w884]
                      tunnel: [refnum<k21> refnum ("task out") w883] -> w841
                      tunnel: [errorcluster {"status"=FALSE, "code"=0, "source"=""} ("error out") w882] -> w840
                      tunnel: [dbl[][] [] ("data") w881] -> w835
                      tunnel: [dbl[] [] ("data") w880] -> w810
                      frame False {
                        (unwired) dbl[][] [] ("data")
                      }
                      frame True {
                        n418 = local read "Track mirror"() -> (w887:bool)
                        n419 = case shown="False" w887 {
                          tunnel: w886 -> [w894 w903]
                          tunnel: w885 -> [w893 w902]
                          tunnel: w884 -> [w892 w901]
                          tunnel: [w891 w900] -> w883
                          tunnel: [w890 w899] -> w882
                          tunnel: [dbl[][] [] ("data") w897] -> w881
                          tunnel: [w888 dbl[] [] ("data")] -> w880
                          frame False {
                            n420 = call-poly <vilib>:"DAQmx Read.vi"("task/channels in"=w894, "number of samples per channel"=w892, "error in"=w893) -> ("task out"=w891:refnum<k21>, "data"=w888:dbl[], "error out"=w890:errorcluster)  [unwired: 10 in]
                          }
                          frame True {
                            n421 = call-poly <vilib>:"DAQmx Read.vi"("task/channels in"=w903, "number of samples per channel"=w901, "error in"=w902) -> ("task out"=w900:refnum<k21>, "data"=w895:dbl[][], "error out"=w899:errorcluster)  [unwired: 10 in]
                            n422 = Multiply(x=w895, y=2.0) -> (x*y=w897:dbl[][])
                          }
                        }
                      }
                    }
                    n423 = Delete From Array(array=w835, length=w828, index (col)=0 ("disabled index (col)")) -> (array with subset deleted=w834:dbl[][])  [unwired: 1 in, 1 out]
                    n424 = Subtract(x=w825, y=w828) -> (x-y=w826:dbl)
                    n425 = Build Array (concatenate)(w834, w833) -> (w827:dbl[][])
                    n426 = Array Subset(array=w827, index (row)=0 ("index"), length (row)=4 ("length"), index (col)=0 ("index"), length (col)=w826) -> (w818:dbl[][])
                    "Mirrors with offset" <- w818
                    n427 = Index Array(array=w818, index (row)=0) -> (element=w821:dbl[])  [unwired: 1 in]
                    n428 = Build Array (concatenate)(w835, w833) -> (→"Mirror position":dbl[][])
                    n429 = Index Array(array=w818, index (row)=1) -> (element=w816:dbl[])  [unwired: 1 in]
                    n430 = Index Array(array=w818, index (row)=3) -> (element=w820:dbl[])  [unwired: 1 in]
                    n431 = Index Array(array=w818, index (row)=2) -> (element=w815:dbl[])  [unwired: 1 in]
                    n432 = Subtract(x=w821, y=w820) -> (x-y=w813:dbl[])
                    n433 = Subtract(x=w816, y=w815) -> (x-y=w814:dbl[])
                    n434 = Square(x=w813) -> (x^2=w812:dbl[])
                    n435 = Multiply(x=w872, y=w873) -> (x*y=w861:u64)
                    n436 = Build Array(w813, w814) -> (→"Mirror error":dbl[][])
                    n437 = call-poly <vilib>:"Mean.vi"("X"=w812) -> ("mean"=→"Standard deviationslow":dbl)  [unwired: 1 out]
                    n438 = Index Array(array=w835, index (row)=1) -> (element=w849:dbl[])  [unwired: 1 in]
                    n439 = Threshold 1D Array(2:0.0 ("threshold y"), 3:w849) -> (0:w850:dbl)  [unwired: 1 in]
                    n440 = local read "Initial sampling rate (Hz)"() -> (w851:dbl)
                    n441 = Subtract(x=w825, y=100.0) -> (x-y=w809:dbl)
                    n442 = local read "Pixel Delay"() -> (w808:dbl)
                    n443 = local read "Soften points"() -> (w804:i32)
                    n444 = Reciprocal(x=w851) -> (1/x=w852:dbl)
                    n445 = Subtract(x=w850, y=w838) -> (x-y=w837:dbl)
                    n446 = Multiply(x=w837, y=w852) -> (x*y=→"Galvo Delay (sec)":dbl)
                    n447 = local read "Scan mode"() -> (w860:T5)
                    n448 = local read "Soften"() -> (w806:bool)
                    n449 = Round To Nearest(number=w837) -> (nearest integer value=→"Delay (pixels)":dbl)
                    n450 = Array Subset(array=w810, index=w808, length=w809) -> (w807:dbl[])
                    n451 = Multiply(x=w804, y=4.0) -> (x*y=w803:dbl)
                    n452 = case shown="\"Single Direction (Uniform)\"" w860 {
                      tunnel: w861 -> [w925 w944 w954 _ _]
                      tunnel: w871 -> [w917 w942 w953 w1012 w1022]
                      tunnel: w870 -> [_ _ w956 w1003 w1020]
                      tunnel: [w923 w941 w955 w1007 w1021] -> w859
                      tunnel: w807 -> [w916 w935 w952 w1006 w1019]
                      tunnel: w806 -> [w915 w934 w951 w1005 _]
                      tunnel: w803 -> [w914 w932 w950 w1004 _]
                      frame "Single Direction (Uniform)" {
                        n453 = Multiply(x=w925, y=u64 2) -> (x*y=w926:u64)
                        n454 = Divide(x=w926, y=w917) -> (x/y=w913:dbl)
                        n455 = case shown="True" w915 {
                          tunnel: w914 -> [_ w930]
                          tunnel: w913 -> [w927 w929]
                          tunnel: [w927 w928] -> w912
                          frame False {
                          }
                          frame True {
                            n456 = Add(x=w929, y=w930) -> (x+y=w928:dbl)
                          }
                        }
                        n457 = Reshape Array(w916, w917, w912) -> (w922:dbl[][])
                        n458 = Divide(x=w913, y=2.0) -> (x/y=w918:dbl)
                        n459 = Array Subset(array=w922, index (row)=0 ("index"), length (row)=w917, index (col)=0 ("index"), length (col)=w918) -> (w923:dbl[][])
                      }
                      frame "Adjustable sawtooth" {
                        n460 = Multiply(x=w944, y=u64 1) -> (x*y=w945:u64)
                        n461 = Divide(x=w945, y=w942) -> (x/y=w933:dbl)
                        n462 = case shown="False" w934 {
                          tunnel: w933 -> [w946 w949]
                          tunnel: w932 -> [_ w948]
                          tunnel: [w946 w947] -> w931
                          frame False {
                          }
                          frame True {
                            n463 = Add(x=w949, y=w948) -> (x+y=w947:dbl)
                          }
                        }
                        n464 = local read "Asymmetry sawtooth"() -> (w937:dbl)
                        n465 = Reshape Array(w935, w942, w931) -> (w940:dbl[][])
                        n466 = Multiply(x=w933, y=w937) -> (x*y=w936:dbl)
                        n467 = Array Subset(array=w940, index (row)=0 ("index"), length (row)=w942, index (col)=0 ("index"), length (col)=w936) -> (w941:dbl[][])
                      }
                      frame "Bi-Directional" {
                        n468 = case shown="True" w951 {
                          tunnel: w956 -> [w958 w999]
                          tunnel: [w979 w998] -> w955
                          tunnel: w954 -> [w978 w997]
                          tunnel: w953 -> [w966 w983]
                          tunnel: w952 -> [w965 w982]
                          tunnel: w950 -> [w962 _]
                          frame True {
                            n469 = Divide(x=w966, y=u16 2) -> (x/y=w971:dbl)
                            n470 = Divide(x=w978, y=w971) -> (x/y=w964:dbl)
                            n471 = Add(x=w964, y=w962) -> (x+y=w963:dbl)
                            n472 = Divide(x=w962, y=2.0) -> (x/y=w960:dbl)
                            n473 = Reshape Array(w965, w971, w963) -> (w972:dbl[][])
                            n474 = Add(x=w958, y=w960) -> (x+y=w957:dbl)
                            n475 = Divide(x=w964, y=2.0) -> (x/y=w959:dbl)
                            n476 = Array Subset(array=w972, index (row)=0 ("index"), length (row)=w971, index (col)=w957, length (col)=w959) -> (w967:dbl[][])
                            n477 = Array Subset(array=w972, index (row)=0 ("index"), length (row)=w971, index (col)=0 ("index"), length (col)=w959) -> (w968:dbl[][])
                            n478 = for {
                              tunnel: w967 -> [w981] mode=indexing
                              tunnel: [w980] -> w970 mode=indexing
                              n479 = Reverse 1D Array(array=w981) -> (reversed array=w980:dbl[])
                            }
                            n480 = Insert Into Array(array=w968, index (col)=w958, new element=w970) -> (w969:dbl[][])  [unwired: 1 in]
                            n481 = Reshape Array(w969, w966, w958) -> (w979:dbl[][])
                          }
                          frame False {
                            n482 = Divide(x=w983, y=u16 2) -> (x/y=w989:dbl)
                            n483 = Divide(x=w997, y=w989) -> (x/y=w995:dbl)
                            n484 = Reshape Array(w982, w989, w995) -> (w990:dbl[][])
                            n485 = Divide(x=w995, y=2.0) -> (x/y=w988:dbl)
                            n486 = Array Subset(array=w990, index (row)=0 ("index"), length (row)=w989, index (col)=w999, length (col)=w988) -> (w984:dbl[][])
                            n487 = Array Subset(array=w990, index (row)=0 ("index"), length (row)=w989, index (col)=0 ("index"), length (col)=w988) -> (w985:dbl[][])
                            n488 = for {
                              tunnel: w984 -> [w1001] mode=indexing
                              tunnel: [w1000] -> w987 mode=indexing
                              n489 = Reverse 1D Array(array=w1001) -> (reversed array=w1000:dbl[])
                            }
                            n490 = Insert Into Array(array=w985, index (col)=w999, new element=w987) -> (w986:dbl[][])  [unwired: 1 in]
                            n491 = Reshape Array(w986, w983, w999) -> (w998:dbl[][])
                          }
                        }
                      }
                      frame "Single Direction (Fast Reset)" {
                        n492 = case shown="True" w1005 {
                          tunnel: w1003 -> [w1015 w1018]
                          tunnel: w1004 -> [_ w1017]
                          tunnel: [w1015 w1016] -> w1002
                          frame False {
                          }
                          frame True {
                            n493 = Add(x=w1018, y=w1017) -> (x+y=w1016:dbl)
                          }
                        }
                        n494 = local read "Xrange"() -> (w1009:u16)
                        n495 = Reshape Array(w1006, w1012, w1002) -> (w1014:dbl[][])
                        n496 = Multiply(x=w1009, y=0.9) -> (x*y=w1008:dbl)
                        n497 = Array Subset(array=w1014, index (row)=0 ("index"), length (row)=w1012, index (col)=0 ("index"), length (col)=w1008) -> (w1007:dbl[][])
                      }
                      frame "Lissajous" {
                        n498 = Reshape Array(w1019, w1022, w1020) -> (w1021:dbl[][])
                      }
                    }
                    n499 = call <vilib>:"DAQmx Is Task Done.vi"("task/channels in"=w841, "error in"=w840) -> ("task out"=w864:refnum<k21>, "task done?"=w867:bool, "error out"=w863:errorcluster)  [unwired: 11 out]
                    n500 = local read "Scan mode"() -> (w857:T5)
                    n501 = Transpose 2D Array(2D array=w859) -> (transposed array=w858:dbl[][])
                    n502 = case shown="\"Single Direction (Fast Reset)\"" w857 {
                      tunnel: w858 -> [w904 w905 w906 w907 w911]
                      tunnel: [w904 w905 w906 w907 w910] -> w869
                      frame "Lissajous" {
                      }
                      frame "Adjustable sawtooth" {
                      }
                      frame "Bi-Directional" {
                      }
                      frame "Single Direction (Uniform)", Default {
                      }
                      frame "Single Direction (Fast Reset)" {
                        n503 = local read "Length to cut"() -> (w909:i32)
                        n504 = local read "Index (col)"() -> (w908:i32)
                        n505 = Delete From Array(array=w911, length=w909, index (row)=w908) -> (array with subset deleted=w910:dbl[][])  [unwired: 1 in, 1 out]
                      }
                    }
                    n506 = property class="DAQmx Read" props=["TotalSampPerChanAcquired", "AvailSampPerChan"](reference=w864, error in=w863) -> (reference out=w875:refnum<k21>, error out=w845:errorcluster, "AvailSampPerChan"=w862:u32)  [unwired: 1 out]
                    n507 = Unbundle By Name(w840) -> ("status"=w865:bool)
                    n508 = Equal To 0?(x=w862) -> (x = 0?=w868:bool)
                    n509 = And(x=w868, y=w867) -> (x .and. y?=w866:bool)
                    n510 = local write "Image (raw)"(w869) -> ()
                    n511 = Wait (ms)(milliseconds to wait=0.05) -> ()  [unwired: 1 out]
                    n512 = Compound Arithmetic op=OR(w865, w854) -> (w874:bool)
                    n513 = Compound Arithmetic op=OR(w866, w865, w854) -> ()  [unwired: 1 out]
                  }
                  frame #2 {
                    n514 = Get Date/Time In Seconds() -> (seconds since 1Jan1904=w1025:timestamp)
                    n515 = Subtract(x=w1025, y=w1024) -> (x-y=w1023:dbl)
                    n516 = local write "Frame rate (s)"(w1023) -> ()
                  }
                }
                n517 = Square(x=w764) -> (x^2=w762:dbl[])
                n518 = call-poly <vilib>:"Mean.vi"("X"=w762) -> ("mean"=→"Standard deviation fast":dbl)  [unwired: 1 out]
              }
            }
            n519 = local read "Frame rate (s)"() -> (w403:dbl)
            n520 = Subtract(x=w386, y=w366) -> (x-y=w402:i32)
            n521 = Multiply(x=w403, y=w402) -> (x*y=w401:dbl)
            n522 = local write "Time left for stack (s)"(w401) -> ()
            n523 = Add Array Elements(numeric array=w384) -> (sum=w382:dbl)
            n524 = Array Size(array=w384) -> (size(s)=w383:i32[])
            n525 = local read "Points/pixel"() -> (w406:u16)
            n526 = To Double Precision Float(number=w383) -> (double precision float=w380:dbl[])
            n527 = Transpose 2D Array(2D array=w407) -> (transposed array=w368:dbl[][])
            n528 = local read "Line scan on/off (raw)"() -> (w371:bool)
            n529 = case shown="True" w371 {
              tunnel: [w543 w546] -> w373
              tunnel: w378 -> [_ w545]
              tunnel: w377 -> [w543 w544]
              frame False {
              }
              frame True {
                n530 = local read "Linecut direction (fast/slow) (raw)"() -> (w549:u8)
                n531 = local read "Linear/Log (raw)"() -> (w548:u16)
                n532 = property on="Image (raw)" class="IntGraph (strict)"() -> ("Cursor.Cursor X"=w551:dbl)  [unwired: 2 in, 2 out]
                n533 = property on="Image (raw)" class="IntGraph (strict)"() -> ("Cursor.Cursor Y"=w550:dbl)  [unwired: 2 in, 2 out]
                n534 = call "Linecut.vi"("linecut y position"=w550, "linecut x position"=w551, "error in (no error)"=w544, "Linear/Log"=w548, "Linecut direction (fast/slow)"=w549, "Input image"=w545) -> ("error out"=w546:errorcluster, "Linecut profile"=w547:dbl[])  [unwired: 4 in]
                n535 = local write "Linecut profile (raw)"(w547) -> ()
              }
            }
            n536 = Multiply Array Elements(1:w380) -> (0:w381:dbl)
            n537 = local read "Average in other dim"() -> (w405:dbl)
            n538 = call "image_avg_no_reshape.vi"("Numeric"=w405, "points / pixel"=w406, "input array"=w368) -> ("output array"=w379:dbl[][])  [unwired: 8 in]
            n539 = Divide(x=w382, y=w381) -> (x/y=w367:dbl)
            n540 = Replace Array Subset(array=w399, new element #1=w398, new element #2=w367) -> (w397:dbl[])  [unwired: 2 in]
            n541 = Transpose 2D Array(2D array=w379) -> (transposed array=w369:dbl[][])
            n542 = local write "Image (integrated)"(w369) -> ()
            n543 = local read "Scan dimension"() -> (w424:T1)
            n544 = local read "Line scan on/off (proccesed)"() -> (w376:bool)
            n545 = case shown="\"XYZ (X: fast, Y: medium, Z: slow)\"" w424 {
              tunnel: w366 -> [w1146 w1151]
              tunnel: w386 -> [_ w1150]
              tunnel: [w1145 w1148] -> w423
              frame "XY (X: fast, Y: slow)", Default {
                n546 = Greater Or Equal?(x=w1146, y=u8 0) -> (x >= y?=w1145:bool)
              }
              frame "XYZ (X: fast, Y: medium, Z: slow)" {
                n547 = Decrement(x=w1150) -> (x-1=w1149:u16)
                n548 = Greater Or Equal?(x=w1151, y=w1149) -> (x >= y?=w1148:bool)
              }
            }
            n549 = local read "# of scans"() -> (w400:u16)
            n550 = case shown="True" w376 {
              tunnel: [w534 w540] -> w372
              tunnel: w375 -> [w534 w537]
              tunnel: w369 -> [_ w536]
              frame False {
              }
              frame True {
                n551 = local read "Linecut direction (fast/slow) (integrated)"() -> (w542:u16)
                n552 = local read "Linear/log (integrated)"() -> (w541:u16)
                n553 = property on="Image (integrated)" class="IntGraph (strict)"() -> ("Cursor.Cursor X"=w535:dbl)  [unwired: 2 in, 2 out]
                n554 = property on="Image (integrated)" class="IntGraph (strict)"() -> ("Cursor.Cursor Y"=w539:dbl)  [unwired: 2 in, 2 out]
                n555 = call "Linecut.vi"("linecut y position"=w539, "linecut x position"=w535, "error in (no error)"=w537, "Linear/Log"=w541, "Linecut direction (fast/slow)"=w542, "Input image"=w536) -> ("error out"=w540:errorcluster, "Linecut profile"=w538:dbl[])  [unwired: 4 in]
                n556 = local write "Linecut profile (integrted)"(w538) -> ()
              }
            }
            n557 = Merge Errors(w373, w372) -> (w374:errorcluster)
            n558 = case shown="1" w400 {
              tunnel: w374 -> [w1032 w1035 w1049]
              tunnel: w369 -> [_ _ w1048]
              tunnel: [path "No scan" ("Appended path") path "Don't  save" ("Appended path") w1047] -> w420
              tunnel: [path "No scan" ("Appended path") path "Don't save" ("Appended path") w1046] -> w385
              tunnel: [w1032 w1035 w1045] -> w358
              tunnel: w407 -> [_ _ w1044]
              frame 0, Default {
              }
              frame 2 {
              }
              frame 1 {
                n559 = local read "Auto-save during single scan (raw)?"() -> (w1043:bool)
                n560 = local read "Auto-save during single scan (integrated)?"() -> (w1042:bool)
                n561 = local read "Rawfile"() -> (w1038:string)
                n562 = local read "Integratedfile"() -> (w1037:string)
                n563 = local read "Save tiff stack (raw)?"() -> (w1036:bool)
                n564 = local read "Save tiff stack (integrated)?"() -> (w1041:bool)
                n565 = call "Save_data.vi"("Data to be saved"=w1044, "Save tiff stack?"=w1036, "File name"=w1038, "Save?"=w1043, "error in (no error)"=w1049) -> ("Appended path"=w1046:path, "error out"=w1039:errorcluster)  [unwired: 9 in]
                n566 = call "Save_data.vi"("Data to be saved"=w1048, "Save tiff stack?"=w1041, "File name"=w1037, "Save?"=w1042, "error in (no error)"=w1049) -> ("Appended path"=w1047:path, "error out"=w1040:errorcluster)  [unwired: 9 in]
                n567 = Merge Errors(w1040, w1039) -> (w1045:errorcluster)
                n568 = local write "Appended path (integrated)"(w1047) -> ()
                n569 = local write "Appended path (raw)"(w1046) -> ()
              }
            }
            n570 = Or(x=w411, y=w423) -> (x .or. y?=w408:bool)
            n571 = call <vilib>:"DAQmx Clear Task.vi"("task in"=w412, "error in"=w358) -> ("error out"=w413:errorcluster)  [unwired: 13 in]
            n572 = call <vilib>:"DAQmx Clear Task.vi"("task in"=w365, "error in"=w413) -> ("error out"=w359:errorcluster)  [unwired: 13 in]
          }
          n573 = Concatenate Strings(w265, w264) -> (w257:string)
          n574 = Or(x=w259, y=w254) -> (x .or. y?=w258:bool)
          n575 = local read "# of scans"() -> (w253:u16)
          n576 = local read "# of scans"() -> (w248:u16)
          n577 = case shown="1" w248 {
            tunnel: w262 -> [w327 w329 w335]
            tunnel: w258 -> [_ w328 _]
            tunnel: [w327 w330 w336] -> w255
            tunnel: w254 -> [_ _ w334]
            frame 0, Default {
            }
            frame 1 {
              n578 = case shown="False" w328 {
                tunnel: w329 -> [w331 w332]
                tunnel: [w331 w332] -> w330
                frame False {
                }
                frame True {
                  n579 = local write "# of scans"(u8 0) -> ()
                }
              }
            }
            frame 2 {
              n580 = case shown="False" w334 {
                tunnel: w335 -> [w337 w338]
                tunnel: [w337 w338] -> w336
                frame False {
                }
                frame True {
                  n581 = local write "# of scans"(u8 0) -> ()
                }
              }
            }
          }
          n582 = case shown="1" w253 {
            tunnel: w266 -> [_ _ w313]
            tunnel: w263 -> [_ _ w305]
            tunnel: w257 -> [_ _ w302]
            tunnel: [w296 w297 w301] -> w256
            tunnel: w255 -> [w296 w297 w300]
            frame 0, Default {
            }
            frame 2 {
            }
            frame 1 {
              # "saving text file"
              n583 = local read "Auto-save during single scan (raw)?"() -> (w309:bool)
              n584 = local read "Auto-save during single scan (integrated)?"() -> (w314:bool)
              n585 = local read "Integratedfile"() -> (w310:string)
              n586 = local read "Rawfile"() -> (w306:string)
              n587 = Search and Replace String(input string=w306, search string=".txt", replace string="_scan_parameters.txt") -> (result string=w299:string)  [unwired: 5 in, 3 out]
              n588 = Search and Replace String(input string=w310, search string=".txt", replace string="_scan_parameters.txt") -> (result string=w298:string)  [unwired: 5 in, 3 out]
              n589 = case shown="True" w314 {
                tunnel: w313 -> [_ w326]
                tunnel: w298 -> [_ w325]
                tunnel: w302 -> [_ w323]
                tunnel: w300 -> [w321 w322]
                tunnel: [w321 w322] -> w303
                frame False {
                }
                frame True {
                  n590 = Build Path(base path=w326, name or relative path=w325) -> (appended path=w324:path)
                  n591 = Write to Text File(file (use dialog)=w324, text=w323) -> ()  [unwired: 2 in, 3 out]
                }
              }
              n592 = case shown="True" w309 {
                tunnel: w305 -> [_ w320]
                tunnel: w299 -> [_ w319]
                tunnel: w302 -> [_ w317]
                tunnel: w300 -> [w315 w316]
                tunnel: [w315 w316] -> w304
                frame False {
                }
                frame True {
                  n593 = Build Path(base path=w320, name or relative path=w319) -> (appended path=w318:path)
                  n594 = Write to Text File(file (use dialog)=w318, text=w317) -> ()  [unwired: 2 in, 3 out]
                }
              }
              n595 = Merge Errors(w303, w304) -> (w301:errorcluster)
            }
          }
        }
      }
      n596 = Add(x="Delay increment", y=w218) -> (x+y=w220:dbl)
    }
    "Delay vs output" <- w192
    n597 = Transpose 2D Array(2D array=w192) -> (transposed array=→"Delay vs output":dbl[][])
  }
  n598 = Unbundle By Name(w12) -> ("VISA resource name"=w19:refnum<visa-resource-name>, "error"=w20:errorcluster)
  n599 = Unbundle By Name(w11) -> ("VISA resource name"=w17:refnum<visa-resource-name>, "error"=w18:errorcluster)
  n600 = Unbundle By Name(w13) -> ("VISA resource name"=w21:refnum<visa-resource-name>, "error"=w22:errorcluster)
  n601 = call "_Close Communications.vi"("Instrument Channel"=w19) -> ()  [unwired: 14 in, 1 out]
  n602 = call <vilib>:"Simple Error Handler.vi"("error in (no error)"=w20) -> ()  [unwired: 1 in, 8 out]
  n603 = call "_Close Communications.vi"("Instrument Channel"=w17) -> ()  [unwired: 14 in, 1 out]
  n604 = call <vilib>:"Simple Error Handler.vi"("error in (no error)"=w18) -> ()  [unwired: 1 in, 8 out]
  n605 = call "_Close Communications.vi"("Instrument Channel"=w21) -> ()  [unwired: 14 in, 1 out]
  n606 = call <vilib>:"Simple Error Handler.vi"("error in (no error)"=w22) -> ()  [unwired: 1 in, 8 out]
  n607 = local write "error out"(w10) -> ()
